vi "3D Experiment Final mouse.vi"() -> ()   [LabVIEW 2011]
uses:
  <vilib>/Utility/miscctls.llb/LV3DPointTypeDef.ctl
  <vilib>/Platform/TimedLoop/XDataNode/timing_clust.ctl
  <vilib>/Platform/TimedLoop/XDataNode/nitl_modes.ctl
  <vilib>/Platform/TimedLoop/XDataNode/wakeup.ctl
  <vilib>/Utility/miscctls.llb/LVRGBAColorTypeDef.ctl
  <vilib>/Utility/inputDevices.llb/closeMouse.vi
  <vilib>/Utility/cursorutil.llb/Set Cursor (Cursor ID).vi
  <vilib>/Utility/inputDevices.llb/mouseAcquire.vi
  <vilib>/Utility/file.llb/Write To Spreadsheet File (DBL).vi
  <vilib>/Utility/file.llb/Write To Spreadsheet File (I64).vi
  <vilib>/Platform/TimedLoop/XDataNode/XDataNode.xnode
  <vilib>/picture/3D Picture Control/NI_3D Picture Control.lvlib
  User32.dll
  <vilib>/Platform/TimedLoop/XDataNode/XDNodeRunTimeDep.lvlib
panel:
  out "initial time 2":u32
  out "initial time":u32
  in  "stop":bool
  out "3D Picture":refnum<vi>(3d-picture)
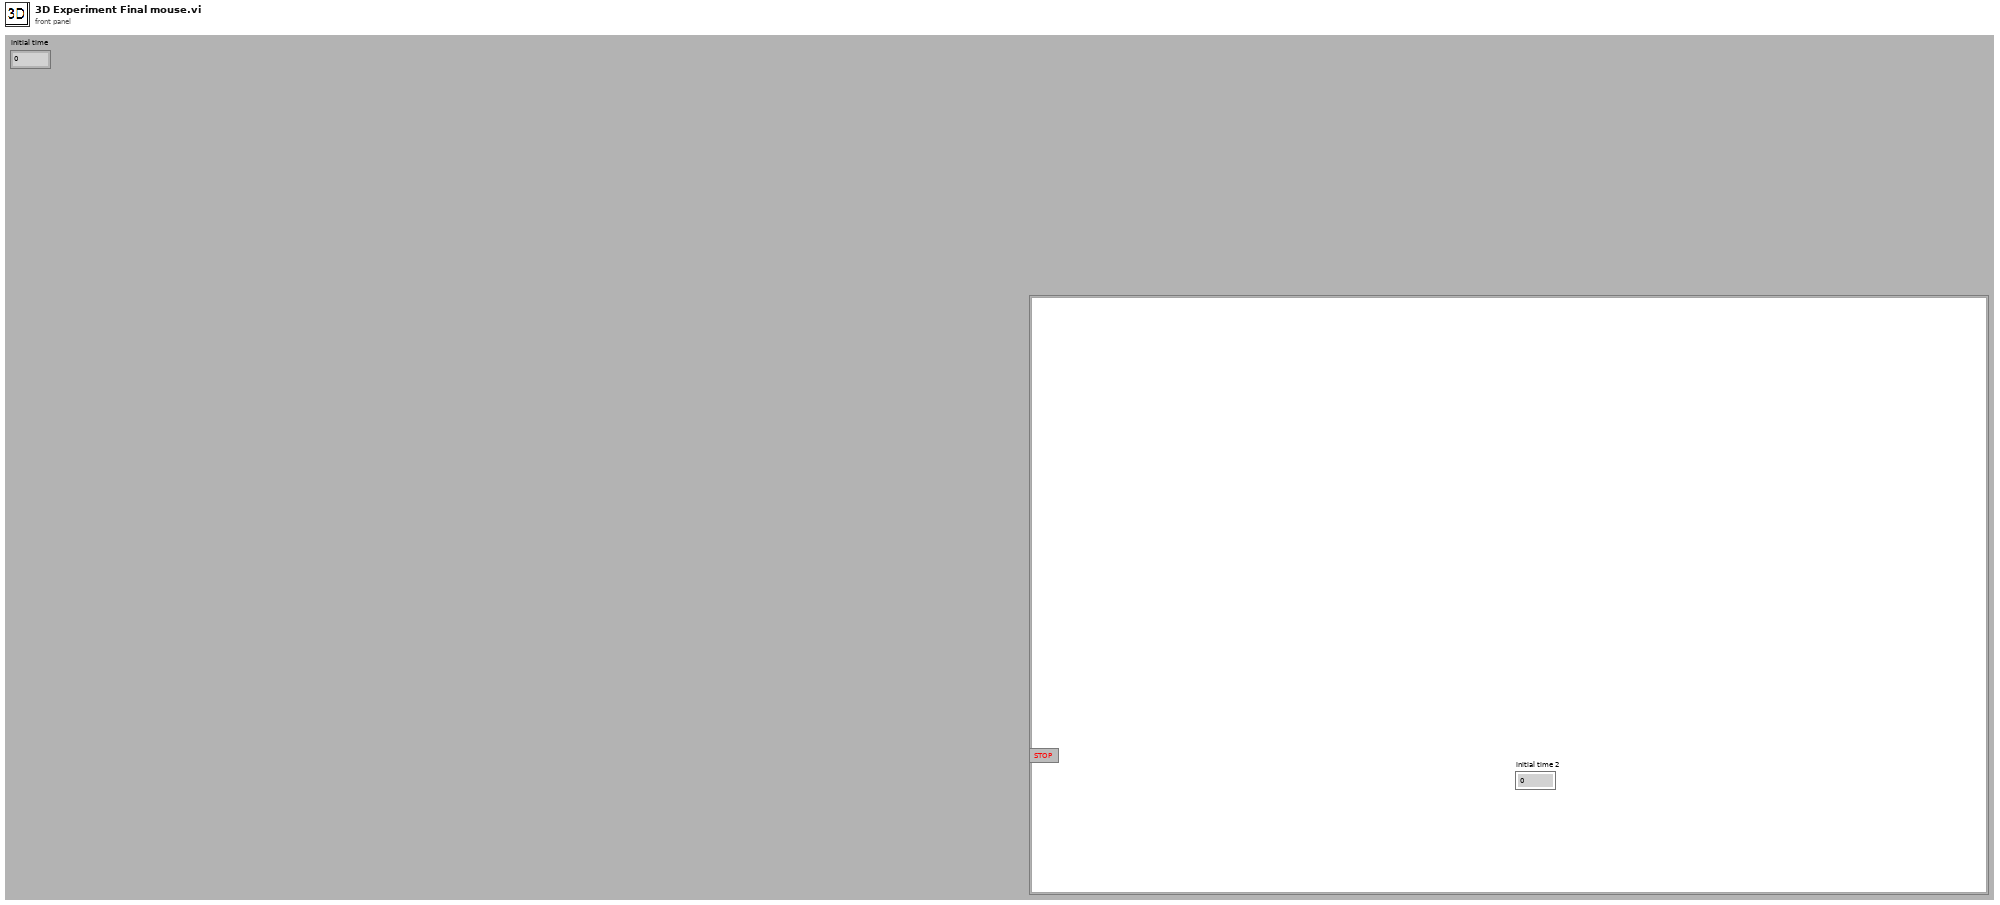
[diagram p1: front panel]
types:
  T1 = enum16{"open", "replace", "create", "open or create", "replace or create", "replace or create with confirmation"}
  T2 = typedef "LV3DPointTypeDef.ctl" = cluster{"X":sgl, "Y":sgl, "Z":sgl}
  T3 = enum16{"Inherit Value", "Points", "Wireframe", "Polygons"}
  T4 = enum16{"Inherit Value", "No Culling", "Cull Back Face", "Cull Front Face", "Cull Both Faces"}
  T5 = enum16{"Zero", "One", "Destination Color", "One Minus Destination Color", "Source Alpha", "One Minus Source Alpha", "Destination Alpha", "One Minus Destination Alpha", "Source Alpha Saturate"}
  T6 = enum16{"Zero", "One", "Source Color", "One Minus Source Color", "Source Alpha", "One Minus Source Alpha", "Destination Alpha", "One Minus Destination Alpha"}
  T7 = enum16{"Normal Bin", "Opaque Bin", "Transparent Bin"}
  T8 = typedef "XDNodeRunTimeDep.lvlib/timing_clust.ctl" = cluster{"Expected End [f-1]":u64, "Actual End [f-1]":u64, "Finished Late? [f-1]":bool, "Expected End [i-1]":u64, "Actual End [i-1]":u64, "Finished Late? [i-1]":bool, "Expected Start [i]":u64, "Actual Start [i]":u64, "Expected Start [f]":u64, "Actual Start [f]":u64, "Source Name":string, "Structure Name":string, "Period":i64, "Deadline":i64, "Offset":i64, "Start":i64, "Priority":i32, "Timeout":i32, "Mode":T9, "Wakeup Reason":T10, "Error":errorcluster, "Source Type":string, "Secondary Source Type":string, "Global End Time":u64, "Global Start Time":u64, "Frame Duration":u64, "Iteration Duration":u64, "Assigned CPU":i32, "I/O Scan Engine Mode":u32}
  T9 = typedef "XDNodeRunTimeDep.lvlib/nitl_modes.ctl" = enum32{"No Change", "Process missed periods, maintain original phase", "Discard missed periods, maintain original phase", "Process missed periods, ignore original phase", "Discard missed periods, ignore original phase"}
  T10 = typedef "XDNodeRunTimeDep.lvlib/wakeup.ctl" = enum32{"Normal", "Aborted", "Asynchronous wakeup", "Timing source error", "Timed loop error", "Timeout"}
  T11 = cluster{"Red":sgl, "Green":sgl, "Blue":sgl, "Alpha":sgl}
  T12 = typedef "LVRGBAColorTypeDef.ctl" = cluster{"Red":sgl, "Green":sgl, "Blue":sgl, "Alpha":sgl}
  T13 = typedef "LVAllMonitorsDisplayTypeDef.ctl" = cluster{"Bounds":cluster{"Left":i16, "Top":i16, "Right":i16, "Bottom":i16}, "Depth":i16}[]
  T14 = cluster{"Bounds":cluster{"Left":i16, "Top":i16, "Right":i16, "Bottom":i16}, "Depth":i16}
  T15 = cluster{"Left":i16, "Top":i16, "Right":i16, "Bottom":i16}
  T16 = cluster{"element":dbl, "Y_scaling":dbl, "element":dbl}
  T17 = cluster{"Horizontal":i32, "Vertical":i32, "Scrolling":i32}
  T18 = cluster{"button 1":bool, "button 2":bool, "button 3":bool, "button 4":bool}
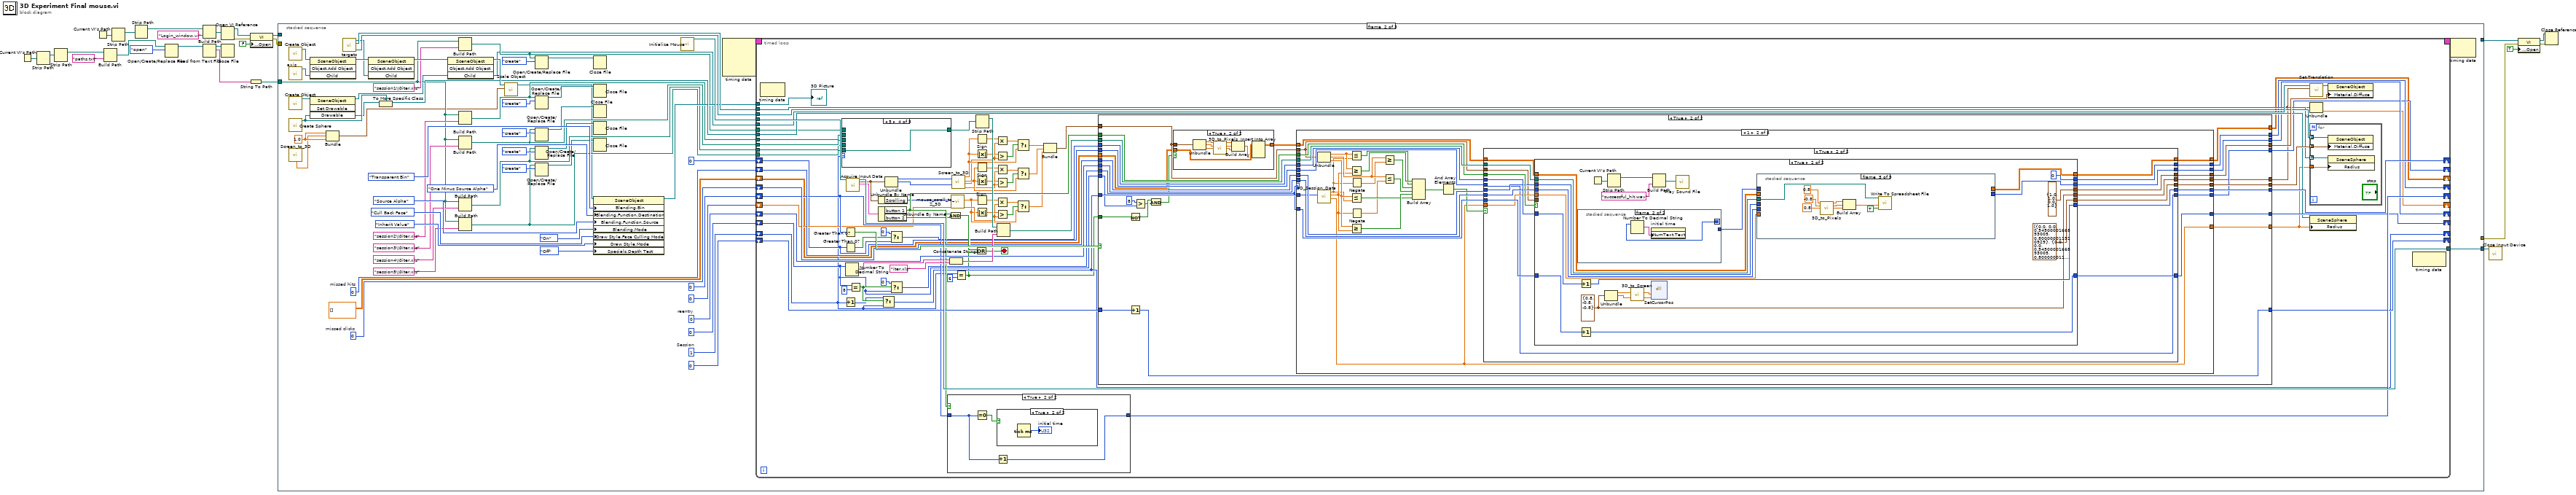
[diagram p0: block diagram]
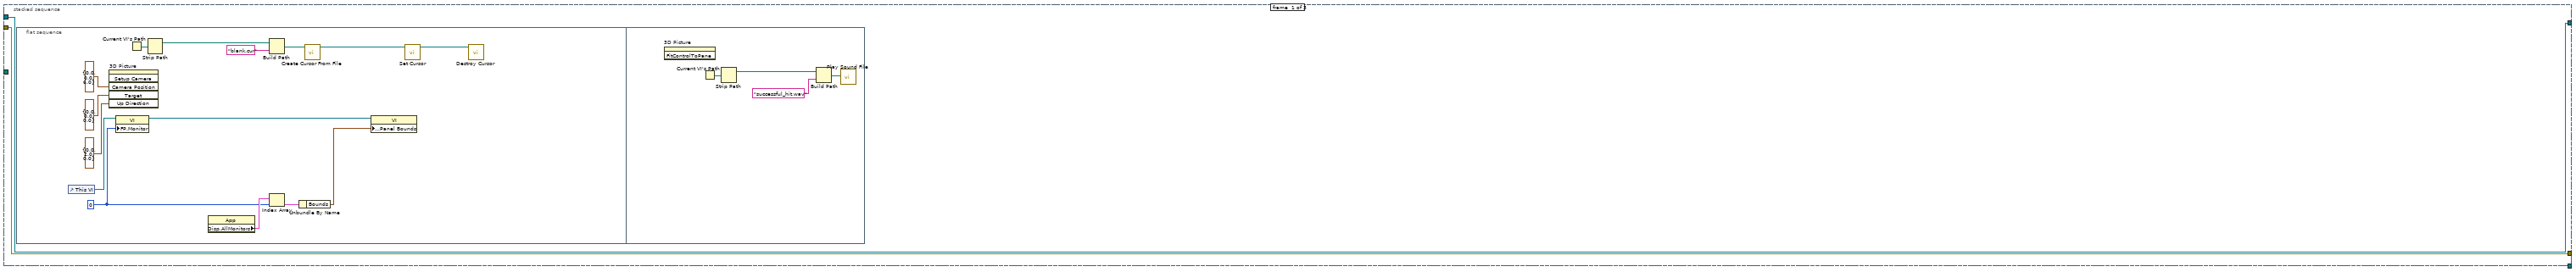
[diagram p2: hidden frame]
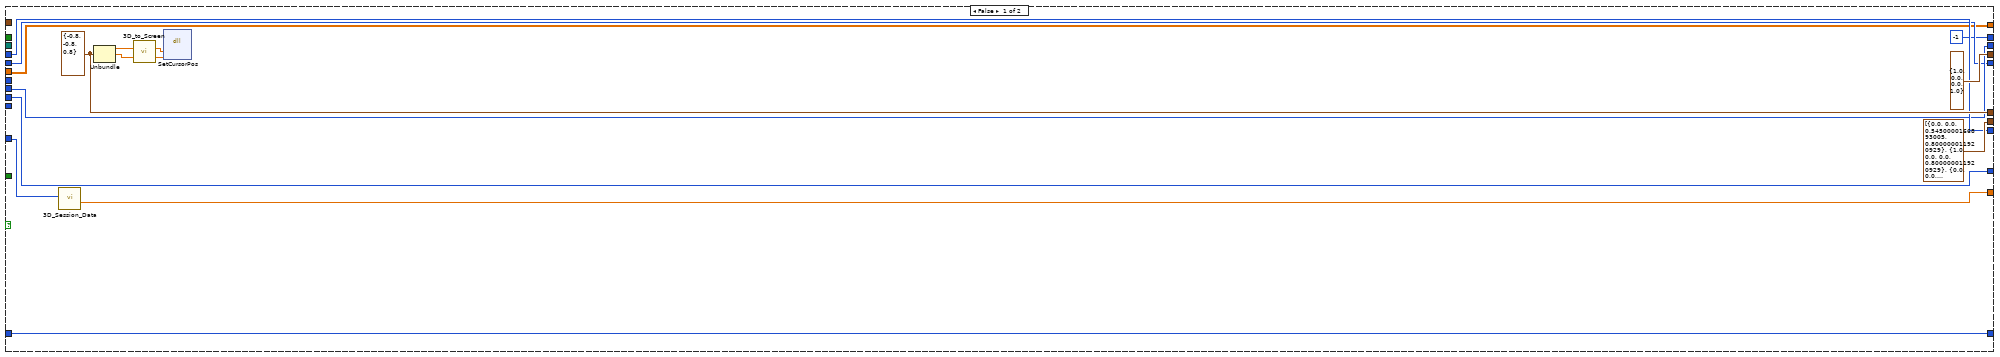
[diagram p7: hidden frame]
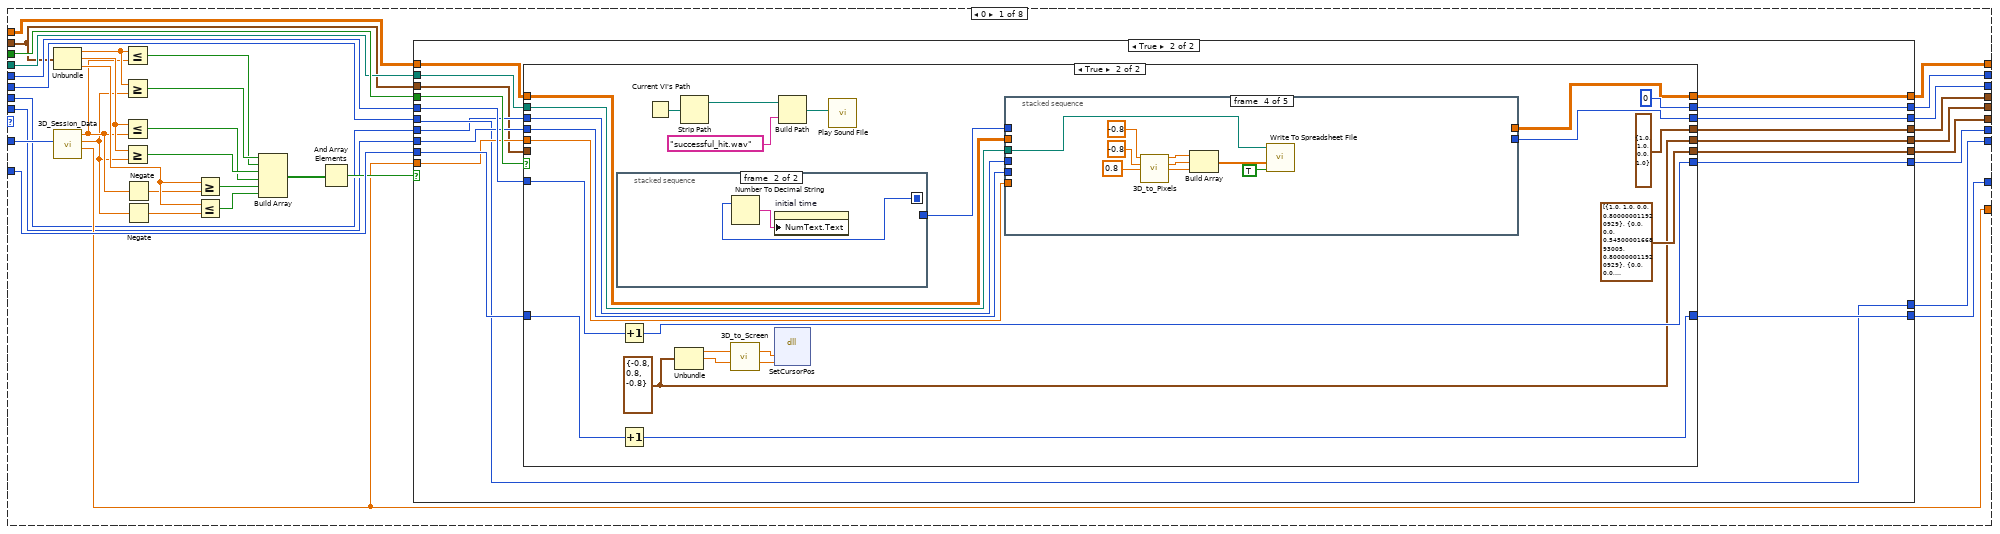
[diagram p9: hidden frame]
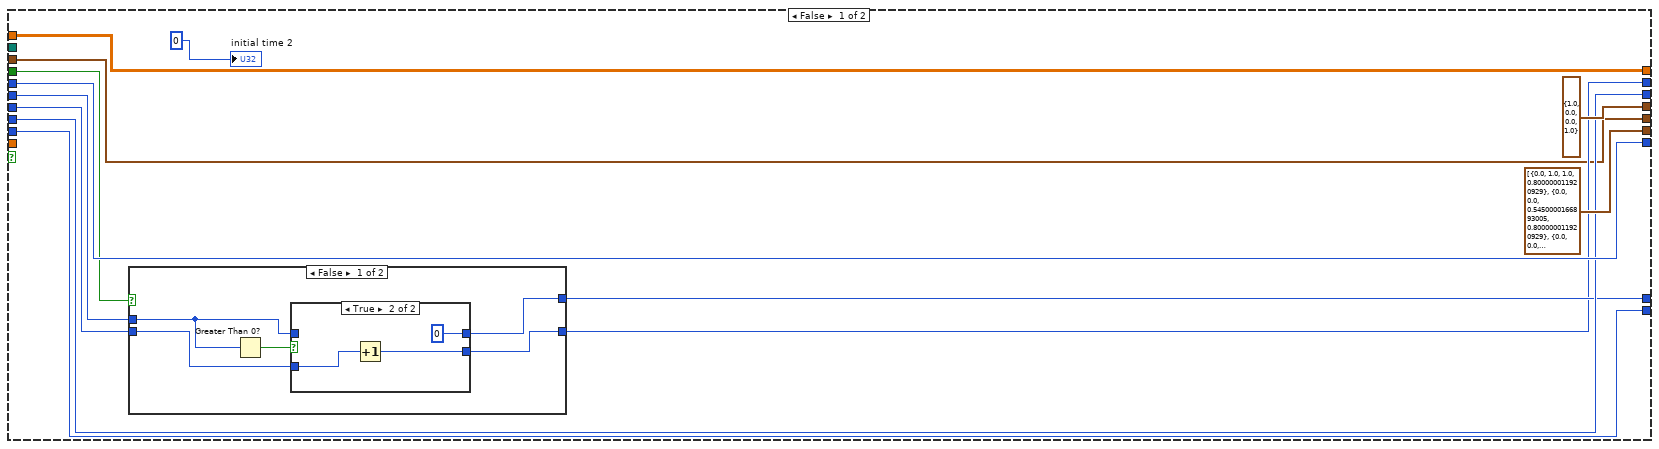
[diagram p10: hidden frame]
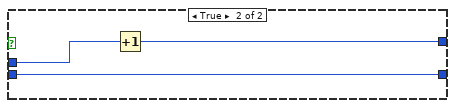
[diagram p12: hidden frame]
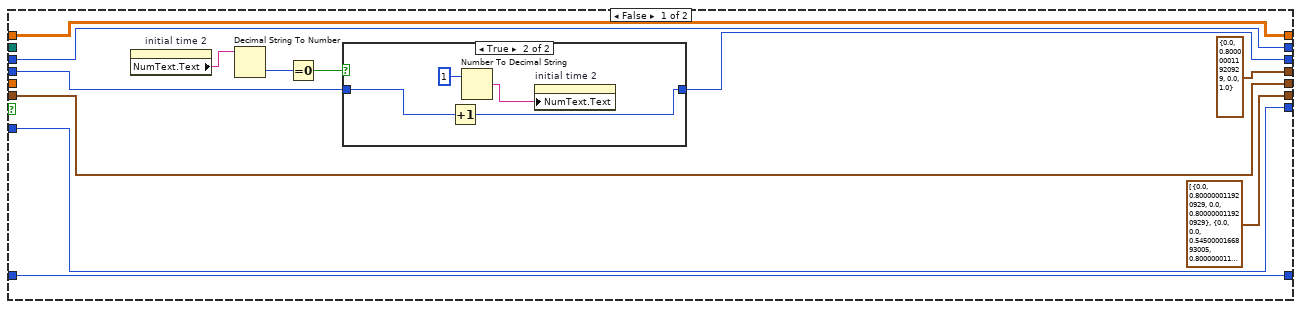
[diagram p13: hidden frame]
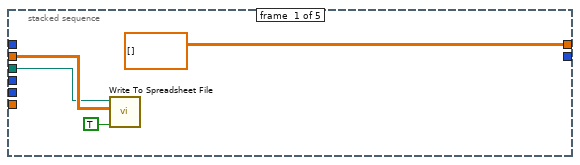
[diagram p15: hidden frame]
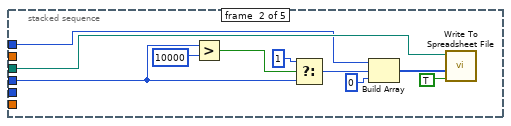
[diagram p16: hidden frame]
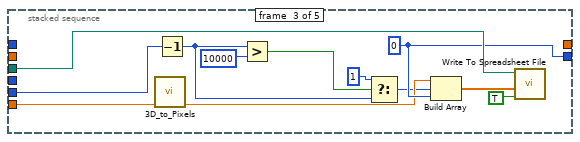
[diagram p17: hidden frame]
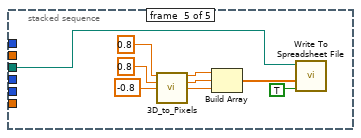
[diagram p18: hidden frame]
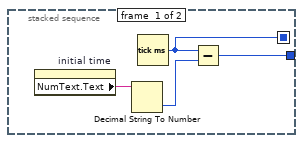
[diagram p19: hidden frame]
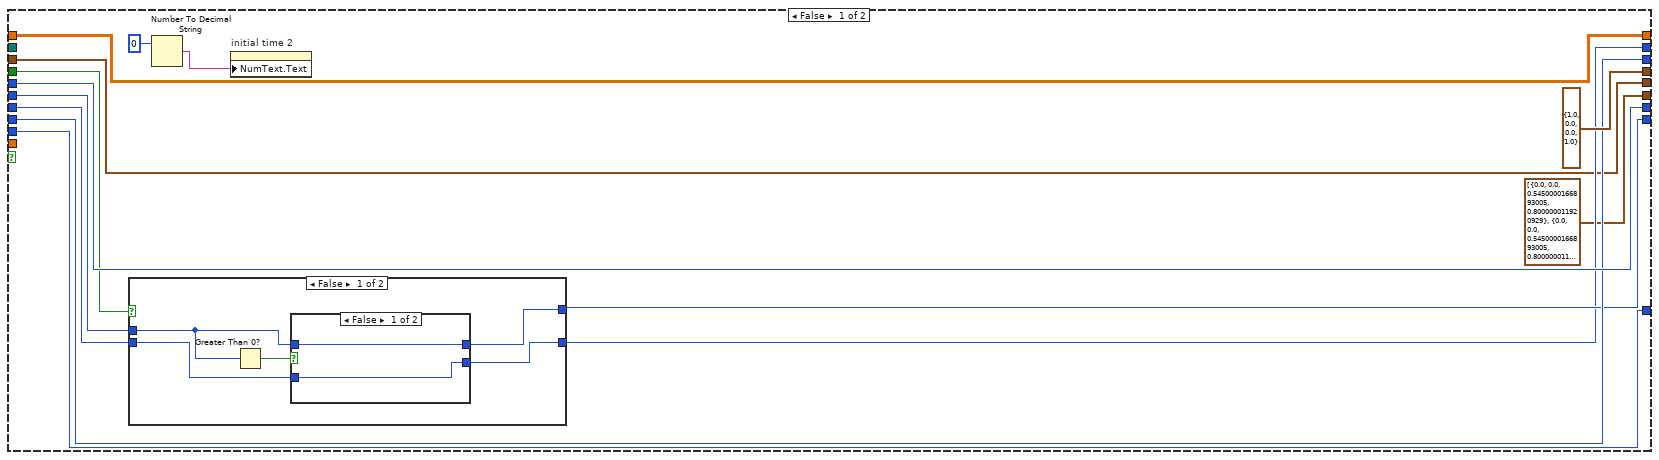
[diagram p20: hidden frame]
diagram:
  n1 = Current VI's Path() -> (path=w1:path)
  n2 = Strip Path(path=w1) -> (stripped path=w2:path)  [unwired: 1 out]
  n3 = Strip Path(path=w2) -> (stripped path=w19:path)  [unwired: 1 out]
  n4 = Current VI's Path() -> (path=w14:path)
  n5 = Build Path(base path=w19, name or relative path="paths.txt") -> (appended path=w22:path)
  n6 = Strip Path(path=w14) -> (stripped path=w11:path)  [unwired: 1 out]
  n7 = Strip Path(path=w11) -> (stripped path=w10:path)  [unwired: 1 out]
  n8 = Open/Create/Replace File(file path (use dialog)=w22, operation (0:open)=T1."open") -> (refnum out=w24:refnum<file>)  [unwired: 4 in, 2 out]
  n9 = Build Path(base path=w10, name or relative path="Login_window.vi") -> (appended path=w12:path)
  n10 = Read from Text File(file (use dialog)=w24) -> (refnum out=w25:refnum<file>, text=w23:string)  [unwired: 3 in, 2 out]
  n11 = Open VI Reference(vi path=w12) -> (vi reference=w17:refnum<vi>, error out=w16:errorcluster)  [unwired: 5 in]
  n12 = Close File(refnum=w25) -> ()  [unwired: 1 in, 2 out]
  n13 = String To Path(string=w23) -> (path=w18:path)
  n14 = property class="VI"(reference=w17, error in=w16, "Front Panel Window:Open"=FALSE) -> (reference out=w9:refnum<vi>, error out=w8:errorcluster)
  n15 = stacked-sequence {
    tunnel: [_ w106 _] -> w26
    tunnel: w18 -> [_ w65 _]
    tunnel: w9 -> [w28 _ _]
    tunnel: w8 -> [w27 _ _]
    tunnel: [w28 _ _] -> w4
    tunnel: [w27 _ _] -> w3
    frame #0 {
      n16 = flat-sequence {
        frame #0 {
          w40 = u16 0 ("Front Panel Window:Monitor")
          n17 = control-ref of="This VI"() -> (w38:refnum<vi>)
          n18 = invoke on="3D Picture" class="SceneGraphDisp (strict)" method="Setup Camera"("Camera Position"=T2 {"X"=0.0, "Y"=0.0, "Z"=6.0}, "Target"=T2 {"X"=0.0, "Y"=0.0, "Z"=0.0}, "Up Direction"=T2 {"X"=0.0, "Y"=2.0, "Z"=0.0}) -> ()  [unwired: 3 in, 6 out]
          n19 = property class="VI"(reference=w38, "FP.Monitor"=w40) -> (reference out=w42:refnum<vi>)  [unwired: 1 in, 1 out]
          n20 = Current VI's Path() -> (path=w37:path)
          n21 = Strip Path(path=w37) -> (stripped path=w36:path)  [unwired: 1 out]
          n22 = property class="App"() -> ("Disp.AllMonitors"=w41:T13)  [unwired: 2 in, 2 out]
          n23 = Build Path(base path=w36, name or relative path="blank.cur") -> (appended path=w34:path)
          n24 = Index Array(array=w41, index=w40) -> (element=w39:T14)
          n25 = Unbundle By Name(w39) -> ("Bounds"=w43:T15)
          n26 = call <vilib>:"Create Cursor From File.vi"("cursor file"=w34) -> ("cursor ID"=w33:refnum<k1>)  [unwired: 9 in, 1 out]
          n27 = property class="VI"(reference=w42, "Front Panel Window:Panel Bounds"=w43) -> ()  [unwired: 1 in, 2 out]
          n28 = call-poly <vilib>:"Set Cursor.vi"("cursor ID"=w33) -> ("previous cursor ID"=w32:refnum<k1>)  [unwired: 9 in, 1 out]
          n29 = call <vilib>:"Destroy Cursor.vi"("cursor ID"=w32) -> ()  [unwired: 9 in, 1 out]
        }
        frame #1 {
          n30 = invoke on="3D Picture" class="SceneGraphDisp (strict)" method="FitControlToPane"() -> ()  [unwired: 3 in, 3 out]
          n31 = Current VI's Path() -> (path=w46:path)
          n32 = Strip Path(path=w46) -> (stripped path=w45:path)  [unwired: 1 out]
          n33 = Build Path(base path=w45, name or relative path="successful_hit.wav") -> (appended path=w47:path)
          n34 = call <vilib>:"Play Sound File.vi"("path"=w47) -> ()  [unwired: 9 in, 2 out]
        }
      }
    }
    frame #1 {
      w52 = 1.0 ("element")
      w53 = 0  # missed clicks
      w54 = 0  # missed hits
      w55 = 0  # reentry
      w94 = 1  # Session
      n35 = call <vilib>:"Create Object.vi"() -> ("Scene:New Object"=w98:refnum<vi>)  [unwired: 10 in, 1 out]
      n36 = call "axis.vi"() -> ("reference out"=w57:refnum<vi>)  [unwired: 11 in]
      n37 = call <vilib>:"Create Object.vi"() -> ("Scene:New Object"=w99:refnum<vi>)  [unwired: 10 in, 1 out]
      n38 = call <vilib>:"Create Sphere.vi"() -> ("New Sphere Refnum"=w92:refnum<vi>)  [unwired: 10 in, 1 out]
      n39 = call "Screen_to_3D.vi"() -> ("Y_scaling"=w49:dbl)  [unwired: 13 in, 6 out]
      n40 = invoke class="SceneObject" method="Object.Add Object"(reference=w98, "Child"=w57) -> (reference out=w97:refnum<vi>)  [unwired: 2 in, 3 out]
      n41 = invoke class="SceneObject" method="Set Drawable"(reference=w99, "Drawable"=w92) -> (reference out=w58:refnum<vi>, "Drawable"=w91:refnum<vi>)  [unwired: 2 in, 2 out]
      n42 = Bundle("element"=w52, "Y_scaling"=w49, "element"=w52) -> (w51:T16)  [unwired: 1 in]
      n43 = call "targets.vi"() -> ("objects"=w93:refnum<vi>[], "shperes"=w89:refnum<vi>[], "Scene:New Object"=w56:refnum<vi>)  [unwired: 8 in]
      n44 = invoke class="SceneObject" method="Object.Add Object"(reference=w97, "Child"=w56) -> (reference out=w96:refnum<vi>)  [unwired: 2 in, 3 out]
      n45 = To More Specific Class(target class=w92, reference=w91) -> (specific class reference=w90:refnum<vi>)  [unwired: 1 in, 1 out]
      n46 = invoke class="SceneObject" method="Object.Add Object"(reference=w96, "Child"=w58) -> (reference out=w95:refnum<vi>, "Child"=w59:refnum<vi>)  [unwired: 2 in, 2 out]
      n47 = Build Path(base path=w65, name or relative path="session1\\0iter.xls") -> (appended path=w60:path)
      n48 = Build Path(base path=w65, name or relative path="session2\\0iter.xls") -> (appended path=w61:path)
      n49 = Build Path(base path=w65, name or relative path="session3\\0iter.xls") -> (appended path=w63:path)
      n50 = Build Path(base path=w65, name or relative path="session4\\0iter.xls") -> (appended path=w62:path)
      n51 = Build Path(base path=w65, name or relative path="session5\\0iter.xls") -> (appended path=w64:path)
      n52 = call <vilib>:"Scale Object.vi"("Scale"=w51, "Scene.Object In"=w95) -> ("Scene.Object Out"=w50:refnum<vi>)  [unwired: 8 in, 1 out]
      n53 = Open/Create/Replace File(file path (use dialog)=w60, operation (0:open)=T1."create") -> (refnum out=w73:refnum<file>)  [unwired: 4 in, 2 out]
      n54 = Open/Create/Replace File(file path (use dialog)=w61, operation (0:open)=T1."create") -> (refnum out=w75:refnum<file>)  [unwired: 4 in, 2 out]
      n55 = Open/Create/Replace File(file path (use dialog)=w63, operation (0:open)=T1."create") -> (refnum out=w70:refnum<file>)  [unwired: 4 in, 2 out]
      n56 = Open/Create/Replace File(file path (use dialog)=w62, operation (0:open)=T1."create") -> (refnum out=w67:refnum<file>)  [unwired: 4 in, 2 out]
      n57 = Open/Create/Replace File(file path (use dialog)=w64, operation (0:open)=T1."create") -> (refnum out=w68:refnum<file>)  [unwired: 4 in, 2 out]
      n58 = Close File(refnum=w73) -> ()  [unwired: 1 in, 2 out]
      n59 = Close File(refnum=w75) -> ()  [unwired: 1 in, 2 out]
      n60 = Close File(refnum=w70) -> ()  [unwired: 1 in, 2 out]
      n61 = Close File(refnum=w67) -> ()  [unwired: 1 in, 2 out]
      n62 = Close File(refnum=w68) -> ()  [unwired: 1 in, 2 out]
      n63 = property class="SceneObject"(reference=w50, "Blending.Bin"=T7."Transparent Bin" ("Blending:Bin"), "Blending.Function.Destination"=T6."One Minus Source Alpha" ("Blending:Function:Destination"), "Blending.Function.Source"=T5."Source Alpha" ("Blending:Function:Source"), "Blending.Mode"=enum16{"Inherit Value", "Off", "On"}."On" ("Blending:Mode"), "Draw Style.Face Culling Mode"=T4."Cull Back Face" ("Draw Style:Face Culling Mode"), "Draw Style.Mode"=T3."Inherit Value" ("Draw Style:Mode"), "Specials.Depth Test"=enum16{"Inherit Value", "Off", "On"}."Off" ("Specials:Depth Test")) -> (reference out=w81:refnum<vi>)  [unwired: 1 in, 1 out]
      n64 = call <vilib>:"Initialize Mouse.vi"() -> ("device ID"=w105:refnum<k1>)  [unwired: 1 in, 10 out]
      n65 = node-c288() -> (w108:T8)  [unwired: 4 in]
      n66 = timed-loop {
        tunnel: [w193] -> w106
        tunnel: w105 -> [w192]
        shift-right: [w191] -> _
        shift-left: 0 ("y") -> [w153]
        shift-right: [w188] -> _
        shift-left: 0 ("y") -> [w137]
        shift-right: [w118] -> _
        shift-left: 0 ("x") -> [w146]
        shift-right: [w186] -> _
        shift-left: 0 ("y") -> [w142]
        timing: w108 -> [_]
        timing-out: [_] -> w107
        shift-right: [w117] -> _
        shift-left: w94 -> [w116]
        shift-right: [w182] -> _
        shift-left: 0 ("y") -> [w183]
        tunnel: w81 -> [w181]
        tunnel: w59 -> [w180]
        tunnel: w93 -> [w177]
        tunnel: w90 -> [w175]
        tunnel: w89 -> [w173]
        tunnel: w64 -> [w169]
        tunnel: w63 -> [w168]
        tunnel: w62 -> [w167]
        tunnel: w61 -> [w166]
        tunnel: w60 -> [w165]
        shift-right: [w160] -> _
        shift-left: w55 -> [w161]
        shift-right: [w154] -> _
        shift-left: w54 -> [w157]
        shift-right: [w155] -> _
        shift-left: w53 -> [w156]
        shift-right: [w113] -> _
        shift-left: dbl[][] [] -> [w114]
        stop <- w158 stop-if-true
        n67 = node-c288() -> ()  [unwired: 1 in, 1 out]
        n68 = case shown="5" w116 {
          tunnel: w169 -> [_ _ _ w197 _]
          tunnel: w167 -> [_ _ w196 _ _]
          tunnel: w168 -> [_ w195 _ _ _]
          tunnel: w166 -> [w194 _ _ _ _]
          tunnel: w165 -> [_ _ _ _ w198]
          tunnel: [w194 w195 w196 w197 w198] -> w162
          frame 2 {
          }
          frame 3 {
          }
          frame 4 {
          }
          frame 5 {
          }
          frame 1, Default {
          }
        }
        n69 = Greater Than 0?(x=w153) -> (x > 0?=w190:bool)
        n70 = Greater Than 0?(x=w142) -> (x > 0?=w145:bool)
        n71 = Increment(x=w116) -> (x+1=w138:i32)
        n72 = Number To Decimal String(number=w137) -> (decimal integer string=w170:string)  [unwired: 1 in]
        n73 = call-poly <vilib>:"Acquire Input Data.vi"("device ID"=w192) -> ("device ID"=w193:refnum<k1>, "axis info"=w187:T17, "button info"=w189:T18)  [unwired: 2 in, 14 out]
        n74 = Equal?(x=w137, y=8) -> (x = y?=w141:bool)
        n75 = Unbundle By Name(w187) -> ("Scrolling"=w147:i32)
        n76 = Unbundle By Name(w189) -> ("button 1"=w152:bool, "button 2"=w151:bool)
        n77 = Select(t=w138, s=w141, f=w116) -> (s? t:f=w117:i32)
        n78 = Unbundle(w187) -> ("Horizontal"=w149:i32, "Vertical"=w148:i32)  [unwired: 1 out]
        n79 = Select(t=0 ("y"), s=w145, f=w142) -> (s? t:f=w143:i32)
        n80 = Select(t=0 ("y"), s=w141, f=w137) -> (s? t:f=w139:i32)
        n81 = case shown="True" w152 {
          tunnel: w153 -> [w1626 w1627]
          tunnel: [w1626 w1629] -> w191
          frame False {
          }
          frame True {
            n82 = Equal To 0?(x=w1627) -> (x = 0?=w1628:bool)
            n83 = Increment(x=w1627) -> (x+1=w1629:i32)
            n84 = case shown="True" w1628 {
              frame False {
              }
              frame True {
                n85 = Tick Count (ms)() -> (millisecond timer value=→"initial time":u32)
              }
            }
          }
        }
        n86 = And(x=w152, y=w151) -> (x .and. y?=w159:bool)
        n87 = Concatenate Strings(w170, "iter.xls" ("name or relative path")) -> (w171:string)
        n88 = call "mouse_scroll_to_Z_3D.vi"("Previous_Z"=w146, "Scrolling"=w147) -> ("Zmax"=w132:dbl, "Z"=w112:dbl)  [unwired: 8 in]
        n89 = call "Screen_to_3D.vi"("X"=w149, "Y"=w148) -> ("X_3D"=w127:dbl, "Y_3D"=w122:dbl, "Xmax"=w120:dbl, "Ymax"=w121:dbl)  [unwired: 11 in, 3 out]
        n90 = Equal?(x=w116, y=6) -> (x = y?=w115:bool)
        n91 = Or(x=w159, y=w115) -> (x .or. y?=w158:bool)
        n92 = Sign(1:w127) -> (0:w129:dbl)
        n93 = Absolute Value(x=w127) -> (abs(x)=w130:dbl)
        n94 = Sign(1:w122) -> (0:w124:dbl)
        n95 = Absolute Value(x=w122) -> (abs(x)=w125:dbl)
        n96 = Sign(1:w112) -> (0:w134:dbl)
        n97 = Absolute Value(x=w112) -> (abs(x)=w135:dbl)
        n98 = Strip Path(path=w162) -> (stripped path=w163:path)  [unwired: 1 out]
        n99 = Multiply(x=w129, y=w120) -> (x*y=w128:dbl)
        n100 = Greater?(x=w130, y=w120) -> (0:w131:bool)
        n101 = Multiply(x=w124, y=w121) -> (x*y=w123:dbl)
        n102 = Greater?(x=w125, y=w121) -> (0:w126:bool)
        n103 = Multiply(x=w134, y=w132) -> (x*y=w133:dbl)
        n104 = Greater?(x=w135, y=w132) -> (0:w136:bool)
        n105 = Build Path(base path=w163, name or relative path=w171) -> (appended path=w164:path)
        n106 = Select(t=w128, s=w131, f=w127) -> (s? t:f=w110:dbl)
        n107 = Select(t=w123, s=w126, f=w122) -> (s? t:f=w109:dbl)
        n108 = Select(t=w133, s=w136, f=w112) -> (s? t:f=w111:dbl)
        n109 = Bundle("X_3D"=w110, "Y_3D"=w109, "Z"=w111) -> (w150:cluster{"X_3D":dbl, "Y_3D":dbl, "Z":dbl})  [unwired: 1 in]
        n110 = case shown="True" w190 {
          tunnel: w150 -> [_ w230]
          tunnel: [w217 w231] -> w119
          tunnel: [T12[] [{"Red"=0.0, "Green"=0.0, "Blue"=0.545, "Alpha"=0.8}, {"Red"=1.0, "Green"=0.0, "Blue"=0.0, "Alpha"=0.8}, {"Red"=0.0, "Green"=0.0, "Blue"=0.545, "Alpha"=0.8}, {"Red"=0.0, "Green"=0.0, "Blue"=0.545, "Alpha"=0.8}, {"Red"=0.0, "Green"=0.0, "Blue"=0.545, "Alpha"=0.8}, {"Red"=0.0, "Green"=0.0, "Blue"=0.545, "Alpha"=0.8}, {"Red"=0.0, "Green"=0.0, "Blue"=0.545, "Alpha"=0.8}, {"Red"=0.0, "Green"=0.0, "Blue"=0.545, "Alpha"=0.8}] ("Array") w249] -> w176
          tunnel: w139 -> [w218 w228]
          tunnel: w152 -> [_ w247]
          tunnel: [T11 {"Red"=1.0, "Green"=0.0, "Blue"=0.0, "Alpha"=1.0} ("Color") w248] -> w179
          tunnel: [w218 w246] -> w188
          tunnel: w143 -> [w216 w245]
          tunnel: [w216 w244] -> w186
          tunnel: w117 -> [w214 w243]
          tunnel: w183 -> [w215 w242]
          tunnel: [w215 w241] -> w182
          tunnel: [w213 w240] -> w174
          tunnel: w164 -> [_ w236]
          tunnel: w161 -> [w212 w239]
          tunnel: [w212 w238] -> w160
          tunnel: w137 -> [_ w237]
          tunnel: w157 -> [w211 w235]
          tunnel: w156 -> [_ w234]
          tunnel: [-1 ("y") w233] -> w155
          tunnel: [w211 w232] -> w154
          tunnel: w115 -> [_ w227]
          tunnel: w114 -> [w205 w223]
          tunnel: [w205 w221] -> w113
          frame False {
            w217 = cluster{dbl, dbl, "y":dbl} {-0.8, -0.8, "y"=0.8}
            n111 = call "3D_Session_Data.vi"("Session"=w214) -> ("Radius"=w213:sgl)  [unwired: 8 in, 2 out]
            n112 = Unbundle(w217) -> (w210:dbl, w209:dbl)  [unwired: 1 out]
            n113 = call "3D_to_Screen.vi"("X_3D"=w210, "Y_3D"=w209) -> ("X"=w208:dbl, "Y"=w207:dbl)  [unwired: 11 in, 1 out]
            n114 = dll-call lib="User32.dll" fn="SetCursorPos"(w208, w207) -> ()  [unwired: 6 in, 2 out]
          }
          frame True {
            n115 = Not(x=w227) -> (.not. x?=w226:bool)
            n116 = Increment(x=w242) -> (x+1=w241:i32)
            n117 = Greater?(x=8 ("y"), y=w237) -> (0:w225:bool)
            n118 = And(x=w226, y=w225) -> (x .and. y?=w224:bool)
            n119 = case shown="True" w224 {
              tunnel: w230 -> [_ w260]
              tunnel: w223 -> [w250 w253]
              tunnel: [w250 w251] -> w222
              frame False {
              }
              frame True {
                n120 = Unbundle(w260) -> ("X_3D"=w259:dbl, "Y_3D"=w258:dbl, "Z"=w257:dbl)
                n121 = call "3D_to_Pixels.vi"("X_3D"=w259, "Y_3D"=w258, "Z_3D"=w257) -> ("X_pixels"=w256:dbl, "Y_pixels"=w255:dbl, "Z_pixels"=w254:dbl)  [unwired: 9 in, 1 out]
                n122 = Build Array(w256, w255, w254) -> (w252:dbl[])
                n123 = Insert Into Array(array=w253, new element=w252) -> (w251:dbl[][])  [unwired: 2 in]
              }
            }
            n124 = case shown="1" w228 {
              tunnel: [w295 w465 w636 w807 w976 w1147 w1318 w1489] -> w249
              tunnel: w230 -> [w264 w433 w604 w775 w945 w1115 w1285 w1457]
              tunnel: [w294 w464 w635 w806 w975 w1146 w1317 w1488] -> w248
              tunnel: w247 -> [w293 w452 w634 w805 w974 w1145 w1316 w1487]
              tunnel: w228 -> [w292 w463 w633 w804 w973 w1144 w1315 w1486]
              tunnel: [w291 w462 w632 w803 w972 w1143 w1314 w1485] -> w246
              tunnel: w245 -> [w279 w461 w631 w802 w971 w1142 w1313 w1484]
              tunnel: [w278 w460 w630 w801 w970 w1141 w1312 w1483] -> w244
              tunnel: w243 -> [w277 w432 w603 w773 w946 w1114 w1286 w1456]
              tunnel: [w271 w431 w602 w776 w944 w1113 w1284 w1455] -> w240
              tunnel: w236 -> [w272 w459 w629 w800 w969 w1140 w1311 w1482]
              tunnel: w239 -> [w269 w457 w627 w798 w967 w1138 w1309 w1481]
              tunnel: [w270 w458 w628 w799 w968 w1139 w1310 w1480] -> w238
              tunnel: w235 -> [w268 w456 w626 w797 w966 w1137 w1308 w1479]
              tunnel: w234 -> [w267 w455 w625 w796 w965 w1136 w1307 w1478]
              tunnel: [w265 w453 w623 w794 w963 w1134 w1305 w1477] -> w233
              tunnel: [w266 w454 w624 w795 w964 w1135 w1306 w1476] -> w232
              tunnel: [w263 w451 w622 w793 w962 w1133 w1304 w1475] -> w231
              tunnel: w222 -> [w262 w449 w621 w792 w961 w1132 w1303 w1474]
              tunnel: [w261 w450 w620 w791 w960 w1131 w1302 w1473] -> w221
              frame 0 {
                n125 = Unbundle(w264) -> ("X_3D"=w290:dbl, "Y_3D"=w289:dbl, "Z"=w288:dbl)
                n126 = call "3D_Session_Data.vi"("Session"=w277) -> ("Radius"=w271:sgl, "min"=w275:dbl, "max"=w276:dbl)  [unwired: 8 in]
                n127 = Less Or Equal?(x=w290, y=w276) -> (x <= y?=w286:bool)
                n128 = Greater Or Equal?(x=w290, y=w275) -> (x >= y?=w287:bool)
                n129 = Less Or Equal?(x=w289, y=w276) -> (x <= y?=w284:bool)
                n130 = Greater Or Equal?(x=w289, y=w275) -> (x >= y?=w285:bool)
                n131 = Negate(x=w276) -> (-x=w274:dbl)
                n132 = Negate(x=w275) -> (-x=w273:dbl)
                n133 = Greater Or Equal?(x=w288, y=w274) -> (x >= y?=w283:bool)
                n134 = Less Or Equal?(x=w288, y=w273) -> (x <= y?=w282:bool)
                n135 = Build Array(w287, w286, w285, w284, w283, w282) -> (w281:bool[])
                n136 = And Array Elements(Boolean array=w281) -> (logical AND=w280:bool)
                n137 = case shown="True" w280 {
                  tunnel: [T12[] [{"Red"=0.0, "Green"=1.0, "Blue"=1.0, "Alpha"=0.8}, {"Red"=0.0, "Green"=0.0, "Blue"=0.545, "Alpha"=0.8}, {"Red"=0.0, "Green"=0.0, "Blue"=0.545, "Alpha"=0.8}, {"Red"=0.0, "Green"=0.0, "Blue"=0.545, "Alpha"=0.8}, {"Red"=0.0, "Green"=0.0, "Blue"=0.545, "Alpha"=0.8}, {"Red"=0.0, "Green"=0.0, "Blue"=0.545, "Alpha"=0.8}, {"Red"=0.0, "Green"=0.0, "Blue"=0.545, "Alpha"=0.8}, {"Red"=0.0, "Green"=0.0, "Blue"=0.545, "Alpha"=0.8}] ("Array") w339] -> w295
                  tunnel: [T11 {"Red"=1.0, "Green"=0.0, "Blue"=0.0, "Alpha"=1.0} ("Color") w338] -> w294
                  tunnel: w293 -> [w298 w337]
                  tunnel: w292 -> [w306 w336]
                  tunnel: [w306 w335] -> w291
                  tunnel: w279 -> [w305 w334]
                  tunnel: [w305 w333] -> w278
                  tunnel: w272 -> [_ w332]
                  tunnel: w271 -> [_ w331]
                  tunnel: [w304 w330] -> w270
                  tunnel: w269 -> [w304 w329]
                  tunnel: w268 -> [w302 w328]
                  tunnel: w267 -> [w301 w327]
                  tunnel: [w300 w328] -> w266
                  tunnel: [w299 w326] -> w265
                  tunnel: w264 -> [w297 w325]
                  tunnel: [w297 w324] -> w263
                  tunnel: w262 -> [w296 w323]
                  tunnel: [w296 w322] -> w261
                  frame False {
                    n138 = case shown="False" w298 {
                      tunnel: w302 -> [w309 w321]
                      tunnel: [w310 w320] -> w300
                      tunnel: w301 -> [w312 w319]
                      tunnel: [w311 w319] -> w299
                      frame False {
                        n139 = Greater Than 0?(x=w309) -> (x > 0?=w313:bool)
                        n140 = case shown="True" w313 {
                          tunnel: w312 -> [w315 w318]
                          tunnel: [w315 w317] -> w311
                          tunnel: w309 -> [w314 _]
                          tunnel: [w314 0 ("y")] -> w310
                          frame False {
                          }
                          frame True {
                            n141 = Increment(x=w318) -> (x+1=w317:i32)
                          }
                        }
                      }
                      frame True {
                        n142 = Increment(x=w321) -> (x+1=w320:i32)
                      }
                    }
                    "initial time 2" <- u32 0 ("initial time 2")
                  }
                  frame True {
                    n143 = case shown="True" w337 {
                      tunnel: [T12[] [{"Red"=0.0, "Green"=0.8, "Blue"=0.0, "Alpha"=0.8}, {"Red"=0.0, "Green"=0.0, "Blue"=0.545, "Alpha"=0.8}, {"Red"=0.0, "Green"=0.0, "Blue"=0.545, "Alpha"=0.8}, {"Red"=0.0, "Green"=0.0, "Blue"=0.545, "Alpha"=0.8}, {"Red"=0.0, "Green"=0.0, "Blue"=0.545, "Alpha"=0.8}, {"Red"=0.0, "Green"=0.0, "Blue"=0.545, "Alpha"=0.8}, {"Red"=0.0, "Green"=0.0, "Blue"=0.545, "Alpha"=0.8}, {"Red"=0.0, "Green"=0.0, "Blue"=0.545, "Alpha"=0.8}] ("Array") T12[] [{"Red"=1.0, "Green"=1.0, "Blue"=0.0, "Alpha"=0.8}, {"Red"=0.0, "Green"=0.0, "Blue"=0.545, "Alpha"=0.8}, {"Red"=0.0, "Green"=0.0, "Blue"=0.545, "Alpha"=0.8}, {"Red"=0.0, "Green"=0.0, "Blue"=0.545, "Alpha"=0.8}, {"Red"=0.0, "Green"=0.0, "Blue"=0.545, "Alpha"=0.8}, {"Red"=0.0, "Green"=0.0, "Blue"=0.545, "Alpha"=0.8}, {"Red"=0.0, "Green"=0.0, "Blue"=0.545, "Alpha"=0.8}, {"Red"=0.0, "Green"=0.0, "Blue"=0.545, "Alpha"=0.8}] ("Array")] -> w339
                      tunnel: [T11 {"Red"=0.0, "Green"=0.8, "Blue"=0.0, "Alpha"=1.0} ("Color") T11 {"Red"=1.0, "Green"=1.0, "Blue"=0.0, "Alpha"=1.0} ("Color")] -> w338
                      tunnel: w336 -> [w349 w378]
                      tunnel: [w349 w377] -> w335
                      tunnel: w334 -> [w348 w360]
                      tunnel: [w348 w376] -> w333
                      tunnel: w332 -> [_ w370]
                      tunnel: w331 -> [_ w369]
                      tunnel: [w343 w368] -> w330
                      tunnel: w329 -> [w344 w367]
                      tunnel: w327 -> [w342 w366]
                      tunnel: [w342 0 ("x")] -> w326
                      tunnel: w325 -> [w341 _]
                      tunnel: [w341 w359] -> w324
                      tunnel: w323 -> [w340 w358]
                      tunnel: [w340 w357] -> w322
                      frame False {
                        n144 = property on="initial time 2" class="DigNum (strict)"() -> ("NumText.Text"=w346:string)  [unwired: 2 in, 2 out]
                        n145 = Decimal String To Number(string=w346) -> (number=w345:i32)  [unwired: 2 in, 1 out]
                        n146 = Equal To 0?(x=w345) -> (x = 0?=w347:bool)
                        n147 = case shown="True" w347 {
                          tunnel: w344 -> [w352 w356]
                          tunnel: [w352 w355] -> w343
                          frame False {
                          }
                          frame True {
                            n148 = Increment(x=w356) -> (x+1=w355:u32)
                            n149 = Number To Decimal String(number=1) -> (decimal integer string=w354:string)  [unwired: 1 in]
                            n150 = property on="initial time 2" class="DigNum (strict)"("NumText.Text"=w354) -> ()  [unwired: 2 in, 2 out]
                          }
                        }
                      }
                      frame True {
                        w359 = cluster{dbl, dbl, "y":dbl} {-0.8, 0.8, "y"=-0.8}
                        n151 = stacked-sequence {
                          seq-local: [w426 _] -> [_ w429]
                          tunnel: [w425 _] -> w371
                          frame #0 {
                            n152 = property on="initial time" class="DigNum (strict)"() -> ("NumText.Text"=w428:string)  [unwired: 2 in, 2 out]
                            n153 = Decimal String To Number(string=w428) -> (number=w427:i32)  [unwired: 2 in, 1 out]
                            n154 = Tick Count (ms)() -> (millisecond timer value=w426:u32)
                            n155 = Subtract(x=w426, y=w427) -> (x-y=w425:u32)
                          }
                          frame #1 {
                            n156 = Number To Decimal String(number=w429) -> (decimal integer string=w430:string)  [unwired: 1 in]
                            n157 = property on="initial time" class="DigNum (strict)"("NumText.Text"=w430) -> ()  [unwired: 2 in, 2 out]
                          }
                        }
                        n158 = Increment(x=w360) -> (x+1=w376:i32)
                        n159 = Increment(x=w378) -> (x+1=w377:i32)
                        n160 = Current VI's Path() -> (path=w374:path)
                        n161 = Unbundle(w359) -> (w364:dbl, w365:dbl)  [unwired: 1 out]
                        n162 = Strip Path(path=w374) -> (stripped path=w373:path)  [unwired: 1 out]
                        n163 = call "3D_to_Screen.vi"("X_3D"=w364, "Y_3D"=w365) -> ("X"=w363:dbl, "Y"=w362:dbl)  [unwired: 11 in, 1 out]
                        n164 = dll-call lib="User32.dll" fn="SetCursorPos"(w363, w362) -> ()  [unwired: 6 in, 2 out]
                        n165 = Build Path(base path=w373, name or relative path="successful_hit.wav") -> (appended path=w375:path)
                        n166 = call <vilib>:"Play Sound File.vi"("path"=w375) -> ()  [unwired: 9 in, 2 out]
                        n167 = stacked-sequence {
                          tunnel: w370 -> [w381 w393 w404 w414 w423]
                          tunnel: w371 -> [_ w391 _ _ _]
                          tunnel: w369 -> [_ _ w401 _ _]
                          tunnel: [_ _ w402 _ _] -> w368
                          tunnel: w367 -> [_ _ w403 _ _]
                          tunnel: w366 -> [_ w387 _ _ _]
                          tunnel: w358 -> [w383 _ _ _ _]
                          tunnel: [dbl[][] [] _ _ _ _] -> w357
                          frame #0 {
                            n168 = call-poly <vilib>:"Write To Spreadsheet File.vi"("append to file? (new file:F)"=TRUE, "2D data"=w383, "file path (dialog if empty)"=w381) -> ()  [unwired: 5 in, 1 out]
                          }
                          frame #1 {
                            n169 = Greater?(x=w387, y=u32 10000 ("element")) -> (0:w389:bool)
                            n170 = Select(t=1, s=w389, f=w387) -> (s? t:f=w385:i32)
                            n171 = Build Array(w391, w385, u32 0 ("element")) -> (w392:u32[])
                            n172 = call-poly <vilib>:"Write To Spreadsheet File.vi"("append to file? (new file:F)"=TRUE, "1D data"=w392, "file path (dialog if empty)"=w393) -> ()  [unwired: 5 in, 1 out]
                          }
                          frame #2 {
                            w402 = u32 0 ("element")
                            n173 = call "3D_to_Pixels.vi"("Distance_3D"=w401) -> ("Distance_pixels"=w400:dbl)  [unwired: 11 in, 3 out]
                            n174 = Decrement(x=w403) -> (x-1=w396:u32)
                            n175 = Greater?(x=w396, y=u32 10000 ("element")) -> (0:w399:bool)
                            n176 = Select(t=1, s=w399, f=w396) -> (s? t:f=w395:u32)
                            n177 = Build Array(w400, w395, w402) -> (w406:dbl[])
                            n178 = call-poly <vilib>:"Write To Spreadsheet File.vi"("append to file? (new file:F)"=TRUE, "1D data"=w406, "file path (dialog if empty)"=w404) -> ()  [unwired: 5 in, 1 out]
                          }
                          frame #3 {
                            n179 = call "3D_to_Pixels.vi"("X_3D"=-0.8 ("element"), "Y_3D"=-0.8 ("element"), "Z_3D"=0.8 ("element")) -> ("X_pixels"=w411:dbl, "Y_pixels"=w412:dbl, "Z_pixels"=w413:dbl)  [unwired: 9 in, 1 out]
                            n180 = Build Array(w411, w412, w413) -> (w410:dbl[])
                            n181 = call-poly <vilib>:"Write To Spreadsheet File.vi"("append to file? (new file:F)"=TRUE, "1D data"=w410, "file path (dialog if empty)"=w414) -> ()  [unwired: 5 in, 1 out]
                          }
                          frame #4 {
                            n182 = call "3D_to_Pixels.vi"("X_3D"=0.8 ("element"), "Y_3D"=0.8 ("element"), "Z_3D"=-0.8 ("element")) -> ("X_pixels"=w420:dbl, "Y_pixels"=w421:dbl, "Z_pixels"=w422:dbl)  [unwired: 9 in, 1 out]
                            n183 = Build Array(w420, w421, w422) -> (w419:dbl[])
                            n184 = call-poly <vilib>:"Write To Spreadsheet File.vi"("append to file? (new file:F)"=TRUE, "1D data"=w419, "file path (dialog if empty)"=w423) -> ()  [unwired: 5 in, 1 out]
                          }
                        }
                      }
                    }
                  }
                }
              }
              frame 1 {
                n185 = Unbundle(w433) -> ("X_3D"=w448:dbl, "Y_3D"=w447:dbl, "Z"=w446:dbl)
                n186 = call "3D_Session_Data.vi"("Session"=w432) -> ("Radius"=w431:sgl, "min"=w436:dbl, "max"=w435:dbl)  [unwired: 8 in]
                n187 = Less Or Equal?(x=w448, y=w435) -> (x <= y?=w444:bool)
                n188 = Greater Or Equal?(x=w448, y=w436) -> (x >= y?=w445:bool)
                n189 = Less Or Equal?(x=w446, y=w435) -> (x <= y?=w440:bool)
                n190 = Greater Or Equal?(x=w446, y=w436) -> (x >= y?=w441:bool)
                n191 = Negate(x=w435) -> (-x=w438:dbl)
                n192 = Negate(x=w436) -> (-x=w437:dbl)
                n193 = Greater Or Equal?(x=w447, y=w438) -> (x >= y?=w443:bool)
                n194 = Less Or Equal?(x=w447, y=w437) -> (x <= y?=w442:bool)
                n195 = Build Array(w445, w444, w443, w442, w441, w440) -> (w439:bool[])
                n196 = And Array Elements(Boolean array=w439) -> (logical AND=w434:bool)
                n197 = case shown="True" w434 {
                  tunnel: [T12[] [{"Red"=0.0, "Green"=0.0, "Blue"=0.545, "Alpha"=0.8}, {"Red"=0.0, "Green"=0.0, "Blue"=0.545, "Alpha"=0.8}, {"Red"=0.0, "Green"=0.0, "Blue"=0.545, "Alpha"=0.8}, {"Red"=0.0, "Green"=0.0, "Blue"=0.545, "Alpha"=0.8}, {"Red"=0.0, "Green"=0.0, "Blue"=0.545, "Alpha"=0.8}, {"Red"=0.0, "Green"=0.0, "Blue"=0.545, "Alpha"=0.8}, {"Red"=0.0, "Green"=0.0, "Blue"=0.545, "Alpha"=0.8}, {"Red"=0.0, "Green"=1.0, "Blue"=1.0, "Alpha"=0.8}] ("Array") w510] -> w465
                  tunnel: [T11 {"Red"=1.0, "Green"=0.0, "Blue"=0.0, "Alpha"=1.0} ("Color") w509] -> w464
                  tunnel: w452 -> [w469 w508]
                  tunnel: w463 -> [w478 w507]
                  tunnel: [w478 w506] -> w462
                  tunnel: w461 -> [w477 w505]
                  tunnel: [w477 w504] -> w460
                  tunnel: w459 -> [_ w503]
                  tunnel: w431 -> [_ w502]
                  tunnel: [w476 w501] -> w458
                  tunnel: w457 -> [w476 w500]
                  tunnel: w456 -> [w473 w497]
                  tunnel: w455 -> [w472 w499]
                  tunnel: [w471 w497] -> w454
                  tunnel: [w470 w498] -> w453
                  tunnel: w433 -> [w468 w496]
                  tunnel: [w468 w495] -> w451
                  tunnel: [w467 w494] -> w450
                  tunnel: w449 -> [w467 w493]
                  frame False {
                    n198 = case shown="False" w469 {
                      tunnel: w473 -> [w480 w492]
                      tunnel: [w481 w491] -> w471
                      tunnel: w472 -> [w483 w490]
                      tunnel: [w482 w490] -> w470
                      frame False {
                        n199 = Greater Than 0?(x=w480) -> (x > 0?=w484:bool)
                        n200 = case shown="False" w484 {
                          tunnel: w483 -> [w486 w489]
                          tunnel: [w486 w488] -> w482
                          tunnel: w480 -> [w485 _]
                          tunnel: [w485 0 ("missed hits")] -> w481
                          frame False {
                          }
                          frame True {
                            n201 = Increment(x=w489) -> (x+1=w488:i32)
                          }
                        }
                      }
                      frame True {
                        n202 = Increment(x=w492) -> (x+1=w491:i32)
                      }
                    }
                    n203 = Number To Decimal String(number=0) -> (decimal integer string=w475:string)  [unwired: 1 in]
                    n204 = property on="initial time 2" class="DigNum (strict)"("NumText.Text"=w475) -> ()  [unwired: 2 in, 2 out]
                  }
                  frame True {
                    n205 = case shown="True" w508 {
                      tunnel: [T12[] [{"Red"=0.0, "Green"=0.0, "Blue"=0.545, "Alpha"=0.8}, {"Red"=0.0, "Green"=0.0, "Blue"=0.545, "Alpha"=0.8}, {"Red"=0.0, "Green"=0.0, "Blue"=0.545, "Alpha"=0.8}, {"Red"=0.0, "Green"=0.0, "Blue"=0.545, "Alpha"=0.8}, {"Red"=0.0, "Green"=0.0, "Blue"=0.545, "Alpha"=0.8}, {"Red"=0.0, "Green"=0.0, "Blue"=0.545, "Alpha"=0.8}, {"Red"=0.0, "Green"=0.0, "Blue"=0.545, "Alpha"=0.8}, {"Red"=0.0, "Green"=0.8, "Blue"=0.0, "Alpha"=0.8}] ("Array") T12[] [{"Red"=0.0, "Green"=0.0, "Blue"=0.545, "Alpha"=0.8}, {"Red"=0.0, "Green"=0.0, "Blue"=0.545, "Alpha"=0.8}, {"Red"=0.0, "Green"=0.0, "Blue"=0.545, "Alpha"=0.8}, {"Red"=0.0, "Green"=0.0, "Blue"=0.545, "Alpha"=0.8}, {"Red"=0.0, "Green"=0.0, "Blue"=0.545, "Alpha"=0.8}, {"Red"=0.0, "Green"=0.0, "Blue"=0.545, "Alpha"=0.8}, {"Red"=0.0, "Green"=0.0, "Blue"=0.545, "Alpha"=0.8}, {"Red"=1.0, "Green"=1.0, "Blue"=0.0, "Alpha"=0.8}] ("Array")] -> w510
                      tunnel: [T11 {"Red"=0.0, "Green"=0.8, "Blue"=0.0, "Alpha"=1.0} ("Color") T11 {"Red"=1.0, "Green"=1.0, "Blue"=0.0, "Alpha"=1.0} ("Color")] -> w509
                      tunnel: w507 -> [w521 w550]
                      tunnel: [w521 w549] -> w506
                      tunnel: w505 -> [w520 w533]
                      tunnel: [w520 w548] -> w504
                      tunnel: w503 -> [_ w543]
                      tunnel: w502 -> [_ w541]
                      tunnel: [w516 w540] -> w501
                      tunnel: w500 -> [w515 w539]
                      tunnel: w499 -> [w514 w532]
                      tunnel: [w514 0 ("x")] -> w498
                      tunnel: w496 -> [w513 _]
                      tunnel: [w513 w531] -> w495
                      tunnel: [w512 w530] -> w494
                      tunnel: w493 -> [w512 w529]
                      frame False {
                        n206 = property on="initial time 2" class="DigNum (strict)"() -> ("NumText.Text"=w518:string)  [unwired: 2 in, 2 out]
                        n207 = Decimal String To Number(string=w518) -> (number=w517:i32)  [unwired: 2 in, 1 out]
                        n208 = Equal To 0?(x=w517) -> (x = 0?=w519:bool)
                        n209 = case shown="False" w519 {
                          tunnel: w515 -> [w523 w527]
                          tunnel: [w523 w526] -> w516
                          frame False {
                          }
                          frame True {
                            n210 = Increment(x=w527) -> (x+1=w526:u32)
                            n211 = Number To Decimal String(number=1) -> (decimal integer string=w525:string)  [unwired: 1 in]
                            n212 = property on="initial time 2" class="DigNum (strict)"("NumText.Text"=w525) -> ()  [unwired: 2 in, 2 out]
                          }
                        }
                      }
                      frame True {
                        w531 = cluster{dbl, dbl, "y":dbl} {0.8, -0.8, "y"=-0.8}
                        n213 = stacked-sequence {
                          seq-local: [w597 _] -> [_ w600]
                          tunnel: [w596 _] -> w542
                          frame #0 {
                            n214 = property on="initial time" class="DigNum (strict)"() -> ("NumText.Text"=w599:string)  [unwired: 2 in, 2 out]
                            n215 = Decimal String To Number(string=w599) -> (number=w598:i32)  [unwired: 2 in, 1 out]
                            n216 = Tick Count (ms)() -> (millisecond timer value=w597:u32)
                            n217 = Subtract(x=w597, y=w598) -> (x-y=w596:u32)
                          }
                          frame #1 {
                            n218 = Number To Decimal String(number=w600) -> (decimal integer string=w601:string)  [unwired: 1 in]
                            n219 = property on="initial time" class="DigNum (strict)"("NumText.Text"=w601) -> ()  [unwired: 2 in, 2 out]
                          }
                        }
                        n220 = Increment(x=w533) -> (x+1=w548:i32)
                        n221 = Increment(x=w550) -> (x+1=w549:i32)
                        n222 = Current VI's Path() -> (path=w546:path)
                        n223 = Unbundle(w531) -> (w537:dbl, w538:dbl)  [unwired: 1 out]
                        n224 = Strip Path(path=w546) -> (stripped path=w545:path)  [unwired: 1 out]
                        n225 = call "3D_to_Screen.vi"("X_3D"=w537, "Y_3D"=w538) -> ("X"=w536:dbl, "Y"=w535:dbl)  [unwired: 11 in, 1 out]
                        n226 = dll-call lib="User32.dll" fn="SetCursorPos"(w536, w535) -> ()  [unwired: 6 in, 2 out]
                        n227 = Build Path(base path=w545, name or relative path="successful_hit.wav") -> (appended path=w547:path)
                        n228 = call <vilib>:"Play Sound File.vi"("path"=w547) -> ()  [unwired: 9 in, 2 out]
                        n229 = stacked-sequence {
                          tunnel: w543 -> [w552 w564 w575 w585 w594]
                          tunnel: w542 -> [_ w562 _ _ _]
                          tunnel: w541 -> [_ _ w572 _ _]
                          tunnel: [_ _ w573 _ _] -> w540
                          tunnel: w539 -> [_ _ w574 _ _]
                          tunnel: w532 -> [_ w557 _ _ _]
                          tunnel: [dbl[][] [] _ _ _ _] -> w530
                          tunnel: w529 -> [w554 _ _ _ _]
                          frame #0 {
                            n230 = call-poly <vilib>:"Write To Spreadsheet File.vi"("append to file? (new file:F)"=TRUE, "2D data"=w554, "file path (dialog if empty)"=w552) -> ()  [unwired: 5 in, 1 out]
                          }
                          frame #1 {
                            n231 = Greater?(x=w557, y=u32 10000 ("element")) -> (0:w560:bool)
                            n232 = Select(t=1, s=w560, f=w557) -> (s? t:f=w556:i32)
                            n233 = Build Array(w562, w556, u32 0 ("element")) -> (w563:u32[])
                            n234 = call-poly <vilib>:"Write To Spreadsheet File.vi"("append to file? (new file:F)"=TRUE, "1D data"=w563, "file path (dialog if empty)"=w564) -> ()  [unwired: 5 in, 1 out]
                          }
                          frame #2 {
                            w573 = u32 0 ("element")
                            n235 = call "3D_to_Pixels.vi"("Distance_3D"=w572) -> ("Distance_pixels"=w571:dbl)  [unwired: 11 in, 3 out]
                            n236 = Decrement(x=w574) -> (x-1=w567:u32)
                            n237 = Greater?(x=w567, y=u32 10000 ("element")) -> (0:w570:bool)
                            n238 = Select(t=1, s=w570, f=w567) -> (s? t:f=w566:u32)
                            n239 = Build Array(w571, w566, w573) -> (w577:dbl[])
                            n240 = call-poly <vilib>:"Write To Spreadsheet File.vi"("append to file? (new file:F)"=TRUE, "1D data"=w577, "file path (dialog if empty)"=w575) -> ()  [unwired: 5 in, 1 out]
                          }
                          frame #3 {
                            n241 = call "3D_to_Pixels.vi"("X_3D"=-0.8 ("element"), "Y_3D"=0.8 ("element"), "Z_3D"=-0.8 ("element")) -> ("X_pixels"=w582:dbl, "Y_pixels"=w583:dbl, "Z_pixels"=w584:dbl)  [unwired: 9 in, 1 out]
                            n242 = Build Array(w582, w583, w584) -> (w581:dbl[])
                            n243 = call-poly <vilib>:"Write To Spreadsheet File.vi"("append to file? (new file:F)"=TRUE, "1D data"=w581, "file path (dialog if empty)"=w585) -> ()  [unwired: 5 in, 1 out]
                          }
                          frame #4 {
                            n244 = call "3D_to_Pixels.vi"("X_3D"=0.8 ("element"), "Y_3D"=-0.8 ("element"), "Z_3D"=0.8 ("element")) -> ("X_pixels"=w593:dbl, "Y_pixels"=w592:dbl, "Z_pixels"=w591:dbl)  [unwired: 9 in, 1 out]
                            n245 = Build Array(w593, w592, w591) -> (w590:dbl[])
                            n246 = call-poly <vilib>:"Write To Spreadsheet File.vi"("append to file? (new file:F)"=TRUE, "1D data"=w590, "file path (dialog if empty)"=w594) -> ()  [unwired: 5 in, 1 out]
                          }
                        }
                      }
                    }
                  }
                }
              }
              frame 2 {
                n247 = Unbundle(w604) -> ("X_3D"=w619:dbl, "Y_3D"=w618:dbl, "Z"=w617:dbl)
                n248 = call "3D_Session_Data.vi"("Session"=w603) -> ("Radius"=w602:sgl, "min"=w607:dbl, "max"=w606:dbl)  [unwired: 8 in]
                n249 = Less Or Equal?(x=w618, y=w606) -> (x <= y?=w613:bool)
                n250 = Greater Or Equal?(x=w618, y=w607) -> (x >= y?=w614:bool)
                n251 = Less Or Equal?(x=w617, y=w606) -> (x <= y?=w611:bool)
                n252 = Greater Or Equal?(x=w617, y=w607) -> (x >= y?=w612:bool)
                n253 = Negate(x=w606) -> (-x=w609:dbl)
                n254 = Negate(x=w607) -> (-x=w608:dbl)
                n255 = Greater Or Equal?(x=w619, y=w609) -> (x >= y?=w616:bool)
                n256 = Less Or Equal?(x=w619, y=w608) -> (x <= y?=w615:bool)
                n257 = Build Array(w616, w615, w614, w613, w612, w611) -> (w610:bool[])
                n258 = And Array Elements(Boolean array=w610) -> (logical AND=w605:bool)
                n259 = case shown="True" w605 {
                  tunnel: [T12[] [{"Red"=0.0, "Green"=0.0, "Blue"=0.545, "Alpha"=0.8}, {"Red"=0.0, "Green"=0.0, "Blue"=0.545, "Alpha"=0.8}, {"Red"=0.0, "Green"=0.0, "Blue"=0.545, "Alpha"=0.8}, {"Red"=0.0, "Green"=0.0, "Blue"=0.545, "Alpha"=0.8}, {"Red"=0.0, "Green"=1.0, "Blue"=1.0, "Alpha"=0.8}, {"Red"=0.0, "Green"=0.0, "Blue"=0.545, "Alpha"=0.8}, {"Red"=0.0, "Green"=0.0, "Blue"=0.545, "Alpha"=0.8}, {"Red"=0.0, "Green"=0.0, "Blue"=0.545, "Alpha"=0.8}] ("Array") w681] -> w636
                  tunnel: [T11 {"Red"=1.0, "Green"=0.0, "Blue"=0.0, "Alpha"=1.0} ("Color") w680] -> w635
                  tunnel: w634 -> [w640 w679]
                  tunnel: w633 -> [w649 w678]
                  tunnel: [w649 w677] -> w632
                  tunnel: w631 -> [w648 w676]
                  tunnel: [w648 w675] -> w630
                  tunnel: w629 -> [_ w674]
                  tunnel: w602 -> [_ w673]
                  tunnel: [w647 w672] -> w628
                  tunnel: w627 -> [w647 w671]
                  tunnel: w626 -> [w644 w668]
                  tunnel: w625 -> [w643 w670]
                  tunnel: [w642 w668] -> w624
                  tunnel: [w641 w669] -> w623
                  tunnel: w604 -> [w639 w667]
                  tunnel: [w639 w666] -> w622
                  tunnel: w621 -> [w638 w665]
                  tunnel: [w638 w664] -> w620
                  frame False {
                    n260 = case shown="True" w640 {
                      tunnel: w644 -> [w651 w663]
                      tunnel: [w652 w662] -> w642
                      tunnel: w643 -> [w654 w661]
                      tunnel: [w653 w661] -> w641
                      frame False {
                        n261 = Greater Than 0?(x=w651) -> (x > 0?=w655:bool)
                        n262 = case shown="False" w655 {
                          tunnel: w654 -> [w657 w660]
                          tunnel: [w657 w659] -> w653
                          tunnel: w651 -> [w656 _]
                          tunnel: [w656 0 ("y")] -> w652
                          frame False {
                          }
                          frame True {
                            n263 = Increment(x=w660) -> (x+1=w659:i32)
                          }
                        }
                      }
                      frame True {
                        n264 = Increment(x=w663) -> (x+1=w662:i32)
                      }
                    }
                    n265 = Number To Decimal String(number=0) -> (decimal integer string=w646:string)  [unwired: 1 in]
                    n266 = property on="initial time 2" class="DigNum (strict)"("NumText.Text"=w646) -> ()  [unwired: 2 in, 2 out]
                  }
                  frame True {
                    n267 = case shown="True" w679 {
                      tunnel: [T12[] [{"Red"=0.0, "Green"=0.0, "Blue"=0.545, "Alpha"=0.8}, {"Red"=0.0, "Green"=0.0, "Blue"=0.545, "Alpha"=0.8}, {"Red"=0.0, "Green"=0.0, "Blue"=0.545, "Alpha"=0.8}, {"Red"=0.0, "Green"=0.0, "Blue"=0.545, "Alpha"=0.8}, {"Red"=0.0, "Green"=0.8, "Blue"=0.0, "Alpha"=0.8}, {"Red"=0.0, "Green"=0.0, "Blue"=0.545, "Alpha"=0.8}, {"Red"=0.0, "Green"=0.0, "Blue"=0.545, "Alpha"=0.8}, {"Red"=0.0, "Green"=0.0, "Blue"=0.545, "Alpha"=0.8}] ("Array") T12[] [{"Red"=0.0, "Green"=0.0, "Blue"=0.545, "Alpha"=0.8}, {"Red"=0.0, "Green"=0.0, "Blue"=0.545, "Alpha"=0.8}, {"Red"=0.0, "Green"=0.0, "Blue"=0.545, "Alpha"=0.8}, {"Red"=0.0, "Green"=0.0, "Blue"=0.545, "Alpha"=0.8}, {"Red"=1.0, "Green"=1.0, "Blue"=0.0, "Alpha"=0.8}, {"Red"=0.0, "Green"=0.0, "Blue"=0.545, "Alpha"=0.8}, {"Red"=0.0, "Green"=0.0, "Blue"=0.545, "Alpha"=0.8}, {"Red"=0.0, "Green"=0.0, "Blue"=0.545, "Alpha"=0.8}] ("Array")] -> w681
                      tunnel: [T11 {"Red"=0.0, "Green"=0.8, "Blue"=0.0, "Alpha"=1.0} ("Color") T11 {"Red"=1.0, "Green"=1.0, "Blue"=0.0, "Alpha"=1.0} ("Color")] -> w680
                      tunnel: w678 -> [w692 w721]
                      tunnel: [w692 w720] -> w677
                      tunnel: w676 -> [w691 w719]
                      tunnel: [w691 w718] -> w675
                      tunnel: w674 -> [_ w712]
                      tunnel: w673 -> [_ w711]
                      tunnel: [w686 w710] -> w672
                      tunnel: w671 -> [w687 w709]
                      tunnel: w670 -> [w685 w708]
                      tunnel: [w685 0 ("missed clicks")] -> w669
                      tunnel: w667 -> [w684 _]
                      tunnel: [w684 w702] -> w666
                      tunnel: w665 -> [w683 w701]
                      tunnel: [w683 w700] -> w664
                      frame False {
                        n268 = property on="initial time 2" class="DigNum (strict)"() -> ("NumText.Text"=w689:string)  [unwired: 2 in, 2 out]
                        n269 = Decimal String To Number(string=w689) -> (number=w688:i32)  [unwired: 2 in, 1 out]
                        n270 = Equal To 0?(x=w688) -> (x = 0?=w690:bool)
                        n271 = case shown="True" w690 {
                          tunnel: w687 -> [w694 w698]
                          tunnel: [w694 w697] -> w686
                          frame False {
                          }
                          frame True {
                            n272 = Increment(x=w698) -> (x+1=w697:u32)
                            n273 = Number To Decimal String(number=1) -> (decimal integer string=w696:string)  [unwired: 1 in]
                            n274 = property on="initial time 2" class="DigNum (strict)"("NumText.Text"=w696) -> ()  [unwired: 2 in, 2 out]
                          }
                        }
                      }
                      frame True {
                        w702 = cluster{dbl, dbl, "y":dbl} {0.8, 0.8, "y"=0.8}
                        n275 = stacked-sequence {
                          seq-local: [w768 _] -> [_ w771]
                          tunnel: [w767 _] -> w713
                          frame #0 {
                            n276 = property on="initial time" class="DigNum (strict)"() -> ("NumText.Text"=w770:string)  [unwired: 2 in, 2 out]
                            n277 = Decimal String To Number(string=w770) -> (number=w769:i32)  [unwired: 2 in, 1 out]
                            n278 = Tick Count (ms)() -> (millisecond timer value=w768:u32)
                            n279 = Subtract(x=w768, y=w769) -> (x-y=w767:u32)
                          }
                          frame #1 {
                            n280 = Number To Decimal String(number=w771) -> (decimal integer string=w772:string)  [unwired: 1 in]
                            n281 = property on="initial time" class="DigNum (strict)"("NumText.Text"=w772) -> ()  [unwired: 2 in, 2 out]
                          }
                        }
                        n282 = Increment(x=w719) -> (x+1=w718:i32)
                        n283 = Increment(x=w721) -> (x+1=w720:i32)
                        n284 = Current VI's Path() -> (path=w716:path)
                        n285 = Unbundle(w702) -> (w707:dbl, w706:dbl)  [unwired: 1 out]
                        n286 = Strip Path(path=w716) -> (stripped path=w715:path)  [unwired: 1 out]
                        n287 = call "3D_to_Screen.vi"("X_3D"=w707, "Y_3D"=w706) -> ("X"=w705:dbl, "Y"=w704:dbl)  [unwired: 11 in, 1 out]
                        n288 = dll-call lib="User32.dll" fn="SetCursorPos"(w705, w704) -> ()  [unwired: 6 in, 2 out]
                        n289 = Build Path(base path=w715, name or relative path="successful_hit.wav") -> (appended path=w717:path)
                        n290 = call <vilib>:"Play Sound File.vi"("path"=w717) -> ()  [unwired: 9 in, 2 out]
                        n291 = stacked-sequence {
                          tunnel: w712 -> [w723 w735 w746 w756 w765]
                          tunnel: w713 -> [_ w733 _ _ _]
                          tunnel: w711 -> [_ _ w742 _ _]
                          tunnel: [_ _ w744 _ _] -> w710
                          tunnel: w709 -> [_ _ w745 _ _]
                          tunnel: w708 -> [_ w728 _ _ _]
                          tunnel: w701 -> [w725 _ _ _ _]
                          tunnel: [dbl[][] [] _ _ _ _] -> w700
                          frame #0 {
                            n292 = call-poly <vilib>:"Write To Spreadsheet File.vi"("append to file? (new file:F)"=TRUE, "2D data"=w725, "file path (dialog if empty)"=w723) -> ()  [unwired: 5 in, 1 out]
                          }
                          frame #1 {
                            n293 = Greater?(x=w728, y=u32 10000 ("element")) -> (0:w731:bool)
                            n294 = Select(t=1, s=w731, f=w728) -> (s? t:f=w727:i32)
                            n295 = Build Array(w733, w727, u32 0 ("element")) -> (w734:u32[])
                            n296 = call-poly <vilib>:"Write To Spreadsheet File.vi"("append to file? (new file:F)"=TRUE, "1D data"=w734, "file path (dialog if empty)"=w735) -> ()  [unwired: 5 in, 1 out]
                          }
                          frame #2 {
                            w744 = u32 0 ("element")
                            n297 = call "3D_to_Pixels.vi"("Distance_3D"=w742) -> ("Distance_pixels"=w743:dbl)  [unwired: 11 in, 3 out]
                            n298 = Decrement(x=w745) -> (x-1=w738:u32)
                            n299 = Greater?(x=w738, y=u32 10000 ("element")) -> (0:w741:bool)
                            n300 = Select(t=1, s=w741, f=w738) -> (s? t:f=w737:u32)
                            n301 = Build Array(w743, w737, w744) -> (w747:dbl[])
                            n302 = call-poly <vilib>:"Write To Spreadsheet File.vi"("append to file? (new file:F)"=TRUE, "1D data"=w747, "file path (dialog if empty)"=w746) -> ()  [unwired: 5 in, 1 out]
                          }
                          frame #3 {
                            n303 = call "3D_to_Pixels.vi"("X_3D"=0.8 ("element"), "Y_3D"=-0.8 ("element"), "Z_3D"=-0.8 ("element")) -> ("X_pixels"=w755:dbl, "Y_pixels"=w754:dbl, "Z_pixels"=w753:dbl)  [unwired: 9 in, 1 out]
                            n304 = Build Array(w755, w754, w753) -> (w752:dbl[])
                            n305 = call-poly <vilib>:"Write To Spreadsheet File.vi"("append to file? (new file:F)"=TRUE, "1D data"=w752, "file path (dialog if empty)"=w756) -> ()  [unwired: 5 in, 1 out]
                          }
                          frame #4 {
                            n306 = call "3D_to_Pixels.vi"("X_3D"=-0.8 ("element"), "Y_3D"=0.8 ("element"), "Z_3D"=0.8 ("element")) -> ("X_pixels"=w764:dbl, "Y_pixels"=w763:dbl, "Z_pixels"=w762:dbl)  [unwired: 9 in, 1 out]
                            n307 = Build Array(w764, w763, w762) -> (w761:dbl[])
                            n308 = call-poly <vilib>:"Write To Spreadsheet File.vi"("append to file? (new file:F)"=TRUE, "1D data"=w761, "file path (dialog if empty)"=w765) -> ()  [unwired: 5 in, 1 out]
                          }
                        }
                      }
                    }
                  }
                }
              }
              frame 3 {
                n309 = call "3D_Session_Data.vi"("Session"=w773) -> ("Radius"=w776:sgl, "min"=w780:dbl, "max"=w774:dbl)  [unwired: 8 in]
                n310 = Unbundle(w775) -> ("X_3D"=w790:dbl, "Y_3D"=w789:dbl, "Z"=w788:dbl)
                n311 = Negate(x=w774) -> (-x=w779:dbl)
                n312 = Negate(x=w780) -> (-x=w778:dbl)
                n313 = Greater Or Equal?(x=w790, y=w779) -> (x >= y?=w787:bool)
                n314 = Greater Or Equal?(x=w789, y=w779) -> (x >= y?=w785:bool)
                n315 = Greater Or Equal?(x=w788, y=w779) -> (x >= y?=w783:bool)
                n316 = Less Or Equal?(x=w790, y=w778) -> (x <= y?=w786:bool)
                n317 = Less Or Equal?(x=w789, y=w778) -> (x <= y?=w784:bool)
                n318 = Less Or Equal?(x=w788, y=w778) -> (x <= y?=w782:bool)
                n319 = Build Array(w787, w786, w785, w784, w783, w782) -> (w781:bool[])
                n320 = And Array Elements(Boolean array=w781) -> (logical AND=w777:bool)
                n321 = case shown="True" w777 {
                  tunnel: [T12[] [{"Red"=0.0, "Green"=0.0, "Blue"=0.545, "Alpha"=0.8}, {"Red"=0.0, "Green"=0.0, "Blue"=0.545, "Alpha"=0.8}, {"Red"=0.0, "Green"=0.0, "Blue"=0.545, "Alpha"=0.8}, {"Red"=0.0, "Green"=1.0, "Blue"=1.0, "Alpha"=0.8}, {"Red"=0.0, "Green"=0.0, "Blue"=0.545, "Alpha"=0.8}, {"Red"=0.0, "Green"=0.0, "Blue"=0.545, "Alpha"=0.8}, {"Red"=0.0, "Green"=0.0, "Blue"=0.545, "Alpha"=0.8}, {"Red"=0.0, "Green"=0.0, "Blue"=0.545, "Alpha"=0.8}] ("Array") w852] -> w807
                  tunnel: [T11 {"Red"=1.0, "Green"=0.0, "Blue"=0.0, "Alpha"=1.0} ("Color") w851] -> w806
                  tunnel: w805 -> [w811 w850]
                  tunnel: w804 -> [w820 w849]
                  tunnel: [w820 w848] -> w803
                  tunnel: w802 -> [w819 w847]
                  tunnel: [w819 w846] -> w801
                  tunnel: w800 -> [_ w845]
                  tunnel: w776 -> [_ w844]
                  tunnel: [w818 w843] -> w799
                  tunnel: w798 -> [w818 w842]
                  tunnel: w797 -> [w815 w841]
                  tunnel: w796 -> [w814 w840]
                  tunnel: [w813 w841] -> w795
                  tunnel: [w812 w839] -> w794
                  tunnel: w775 -> [w810 w838]
                  tunnel: [w810 w837] -> w793
                  tunnel: w792 -> [w809 w836]
                  tunnel: [w809 w835] -> w791
                  frame False {
                    n322 = case shown="False" w811 {
                      tunnel: w815 -> [w823 w834]
                      tunnel: [w822 w833] -> w813
                      tunnel: w814 -> [w825 w832]
                      tunnel: [w824 w832] -> w812
                      frame False {
                        n323 = Equal To 0?(x=w823) -> (x = 0?=w826:bool)
                        n324 = case shown="True" w826 {
                          tunnel: w825 -> [w828 w831]
                          tunnel: [w828 w830] -> w824
                          tunnel: w823 -> [w827 _]
                          tunnel: [w827 0 ("y")] -> w822
                          frame False {
                          }
                          frame True {
                            n325 = Increment(x=w831) -> (x+1=w830:i32)
                          }
                        }
                      }
                      frame True {
                        n326 = Increment(x=w834) -> (x+1=w833:i32)
                      }
                    }
                    n327 = Number To Decimal String(number=0) -> (decimal integer string=w817:string)  [unwired: 1 in]
                    n328 = property on="initial time 2" class="DigNum (strict)"("NumText.Text"=w817) -> ()  [unwired: 2 in, 2 out]
                  }
                  frame True {
                    n329 = case shown="True" w850 {
                      tunnel: [T12[] [{"Red"=0.0, "Green"=0.0, "Blue"=0.545, "Alpha"=0.8}, {"Red"=0.0, "Green"=0.0, "Blue"=0.545, "Alpha"=0.8}, {"Red"=0.0, "Green"=0.0, "Blue"=0.545, "Alpha"=0.8}, {"Red"=0.0, "Green"=0.8, "Blue"=0.0, "Alpha"=0.8}, {"Red"=0.0, "Green"=0.0, "Blue"=0.545, "Alpha"=0.8}, {"Red"=0.0, "Green"=0.0, "Blue"=0.545, "Alpha"=0.8}, {"Red"=0.0, "Green"=0.0, "Blue"=0.545, "Alpha"=0.8}, {"Red"=0.0, "Green"=0.0, "Blue"=0.545, "Alpha"=0.8}] ("Array") T12[] [{"Red"=0.0, "Green"=0.0, "Blue"=0.545, "Alpha"=0.8}, {"Red"=0.0, "Green"=0.0, "Blue"=0.545, "Alpha"=0.8}, {"Red"=0.0, "Green"=0.0, "Blue"=0.545, "Alpha"=0.8}, {"Red"=1.0, "Green"=1.0, "Blue"=0.0, "Alpha"=0.8}, {"Red"=0.0, "Green"=0.0, "Blue"=0.545, "Alpha"=0.8}, {"Red"=0.0, "Green"=0.0, "Blue"=0.545, "Alpha"=0.8}, {"Red"=0.0, "Green"=0.0, "Blue"=0.545, "Alpha"=0.8}, {"Red"=0.0, "Green"=0.0, "Blue"=0.545, "Alpha"=0.8}] ("Array")] -> w852
                      tunnel: [T11 {"Red"=0.0, "Green"=0.8, "Blue"=0.0, "Alpha"=1.0} ("Color") T11 {"Red"=1.0, "Green"=1.0, "Blue"=0.0, "Alpha"=1.0} ("Color")] -> w851
                      tunnel: w849 -> [w863 w892]
                      tunnel: [w863 w891] -> w848
                      tunnel: w847 -> [w862 w890]
                      tunnel: [w862 w889] -> w846
                      tunnel: w845 -> [_ w883]
                      tunnel: w844 -> [_ w882]
                      tunnel: [w857 w881] -> w843
                      tunnel: w842 -> [w858 w880]
                      tunnel: w840 -> [w856 w879]
                      tunnel: [w856 0 ("y")] -> w839
                      tunnel: w838 -> [w855 _]
                      tunnel: [w855 w873] -> w837
                      tunnel: w836 -> [w854 w872]
                      tunnel: [w854 w871] -> w835
                      frame False {
                        n330 = property on="initial time 2" class="DigNum (strict)"() -> ("NumText.Text"=w860:string)  [unwired: 2 in, 2 out]
                        n331 = Decimal String To Number(string=w860) -> (number=w859:i32)  [unwired: 2 in, 1 out]
                        n332 = Equal To 0?(x=w859) -> (x = 0?=w861:bool)
                        n333 = case shown="False" w861 {
                          tunnel: w858 -> [w865 w869]
                          tunnel: [w865 w868] -> w857
                          frame False {
                          }
                          frame True {
                            n334 = Increment(x=w869) -> (x+1=w868:u32)
                            n335 = Number To Decimal String(number=1) -> (decimal integer string=w867:string)  [unwired: 1 in]
                            n336 = property on="initial time 2" class="DigNum (strict)"("NumText.Text"=w867) -> ()  [unwired: 2 in, 2 out]
                          }
                        }
                      }
                      frame True {
                        w873 = cluster{dbl, dbl, "y":dbl} {-0.8, -0.8, "y"=-0.8}
                        n337 = stacked-sequence {
                          seq-local: [w939 _] -> [_ w942]
                          tunnel: [w938 _] -> w884
                          frame #0 {
                            n338 = property on="initial time" class="DigNum (strict)"() -> ("NumText.Text"=w941:string)  [unwired: 2 in, 2 out]
                            n339 = Decimal String To Number(string=w941) -> (number=w940:i32)  [unwired: 2 in, 1 out]
                            n340 = Tick Count (ms)() -> (millisecond timer value=w939:u32)
                            n341 = Subtract(x=w939, y=w940) -> (x-y=w938:u32)
                          }
                          frame #1 {
                            n342 = Number To Decimal String(number=w942) -> (decimal integer string=w943:string)  [unwired: 1 in]
                            n343 = property on="initial time" class="DigNum (strict)"("NumText.Text"=w943) -> ()  [unwired: 2 in, 2 out]
                          }
                        }
                        n344 = Increment(x=w890) -> (x+1=w889:i32)
                        n345 = Increment(x=w892) -> (x+1=w891:i32)
                        n346 = Current VI's Path() -> (path=w887:path)
                        n347 = Unbundle(w873) -> (w878:dbl, w877:dbl)  [unwired: 1 out]
                        n348 = Strip Path(path=w887) -> (stripped path=w886:path)  [unwired: 1 out]
                        n349 = call "3D_to_Screen.vi"("X_3D"=w878, "Y_3D"=w877) -> ("X"=w876:dbl, "Y"=w875:dbl)  [unwired: 11 in, 1 out]
                        n350 = dll-call lib="User32.dll" fn="SetCursorPos"(w876, w875) -> ()  [unwired: 6 in, 2 out]
                        n351 = Build Path(base path=w886, name or relative path="successful_hit.wav") -> (appended path=w888:path)
                        n352 = call <vilib>:"Play Sound File.vi"("path"=w888) -> ()  [unwired: 9 in, 2 out]
                        n353 = stacked-sequence {
                          tunnel: w883 -> [w894 w906 w917 w927 w936]
                          tunnel: w884 -> [_ w904 _ _ _]
                          tunnel: w882 -> [_ _ w914 _ _]
                          tunnel: [_ _ w915 _ _] -> w881
                          tunnel: w880 -> [_ _ w916 _ _]
                          tunnel: w879 -> [_ w899 _ _ _]
                          tunnel: w872 -> [w895 _ _ _ _]
                          tunnel: [dbl[][] [] _ _ _ _] -> w871
                          frame #0 {
                            n354 = call-poly <vilib>:"Write To Spreadsheet File.vi"("append to file? (new file:F)"=TRUE, "2D data"=w895, "file path (dialog if empty)"=w894) -> ()  [unwired: 5 in, 1 out]
                          }
                          frame #1 {
                            n355 = Greater?(x=w899, y=u32 10000 ("element")) -> (0:w902:bool)
                            n356 = Select(t=1, s=w902, f=w899) -> (s? t:f=w898:i32)
                            n357 = Build Array(w904, w898, u32 0 ("element")) -> (w905:u32[])
                            n358 = call-poly <vilib>:"Write To Spreadsheet File.vi"("append to file? (new file:F)"=TRUE, "1D data"=w905, "file path (dialog if empty)"=w906) -> ()  [unwired: 5 in, 1 out]
                          }
                          frame #2 {
                            w915 = u32 0 ("element")
                            n359 = call "3D_to_Pixels.vi"("Distance_3D"=w914) -> ("Distance_pixels"=w913:dbl)  [unwired: 11 in, 3 out]
                            n360 = Decrement(x=w916) -> (x-1=w909:u32)
                            n361 = Greater?(x=w909, y=u32 10000 ("element")) -> (0:w912:bool)
                            n362 = Select(t=1, s=w912, f=w909) -> (s? t:f=w908:u32)
                            n363 = Build Array(w913, w908, w915) -> (w918:dbl[])
                            n364 = call-poly <vilib>:"Write To Spreadsheet File.vi"("append to file? (new file:F)"=TRUE, "1D data"=w918, "file path (dialog if empty)"=w917) -> ()  [unwired: 5 in, 1 out]
                          }
                          frame #3 {
                            n365 = call "3D_to_Pixels.vi"("X_3D"=0.8 ("element"), "Y_3D"=0.8 ("element"), "Z_3D"=0.8 ("element")) -> ("X_pixels"=w926:dbl, "Y_pixels"=w925:dbl, "Z_pixels"=w924:dbl)  [unwired: 9 in, 1 out]
                            n366 = Build Array(w926, w925, w924) -> (w923:dbl[])
                            n367 = call-poly <vilib>:"Write To Spreadsheet File.vi"("append to file? (new file:F)"=TRUE, "1D data"=w923, "file path (dialog if empty)"=w927) -> ()  [unwired: 5 in, 1 out]
                          }
                          frame #4 {
                            n368 = call "3D_to_Pixels.vi"("X_3D"=-0.8 ("element"), "Y_3D"=-0.8 ("element"), "Z_3D"=-0.8 ("element")) -> ("X_pixels"=w935:dbl, "Y_pixels"=w934:dbl, "Z_pixels"=w933:dbl)  [unwired: 9 in, 1 out]
                            n369 = Build Array(w935, w934, w933) -> (w929:dbl[])
                            n370 = call-poly <vilib>:"Write To Spreadsheet File.vi"("append to file? (new file:F)"=TRUE, "1D data"=w929, "file path (dialog if empty)"=w936) -> ()  [unwired: 5 in, 1 out]
                          }
                        }
                      }
                    }
                  }
                }
              }
              frame 4 {
                n371 = Unbundle(w945) -> ("X_3D"=w959:dbl, "Y_3D"=w958:dbl, "Z"=w957:dbl)
                n372 = call "3D_Session_Data.vi"("Session"=w946) -> ("Radius"=w944:sgl, "min"=w949:dbl, "max"=w948:dbl)  [unwired: 8 in]
                n373 = Less Or Equal?(x=w959, y=w948) -> (x <= y?=w955:bool)
                n374 = Greater Or Equal?(x=w959, y=w949) -> (x >= y?=w956:bool)
                n375 = Less Or Equal?(x=w958, y=w948) -> (x <= y?=w953:bool)
                n376 = Greater Or Equal?(x=w958, y=w949) -> (x >= y?=w954:bool)
                n377 = Less Or Equal?(x=w957, y=w948) -> (x <= y?=w951:bool)
                n378 = Greater Or Equal?(x=w957, y=w949) -> (x >= y?=w952:bool)
                n379 = Build Array(w956, w955, w954, w953, w952, w951) -> (w950:bool[])
                n380 = And Array Elements(Boolean array=w950) -> (logical AND=w947:bool)
                n381 = case shown="True" w947 {
                  tunnel: [T12[] [{"Red"=0.0, "Green"=0.0, "Blue"=0.545, "Alpha"=0.8}, {"Red"=0.0, "Green"=0.0, "Blue"=0.545, "Alpha"=0.8}, {"Red"=0.0, "Green"=1.0, "Blue"=1.0, "Alpha"=0.8}, {"Red"=0.0, "Green"=0.0, "Blue"=0.545, "Alpha"=0.8}, {"Red"=0.0, "Green"=0.0, "Blue"=0.545, "Alpha"=0.8}, {"Red"=0.0, "Green"=0.0, "Blue"=0.545, "Alpha"=0.8}, {"Red"=0.0, "Green"=0.0, "Blue"=0.545, "Alpha"=0.8}, {"Red"=0.0, "Green"=0.0, "Blue"=0.545, "Alpha"=0.8}] ("Array") w1021] -> w976
                  tunnel: [T11 {"Red"=1.0, "Green"=0.0, "Blue"=0.0, "Alpha"=1.0} ("Color") w1020] -> w975
                  tunnel: w974 -> [w980 w1019]
                  tunnel: w973 -> [w989 w1018]
                  tunnel: [w989 w1017] -> w972
                  tunnel: w971 -> [w988 w1016]
                  tunnel: [w988 w1015] -> w970
                  tunnel: w969 -> [_ w1014]
                  tunnel: w944 -> [_ w1013]
                  tunnel: [w987 w1011] -> w968
                  tunnel: w967 -> [w987 w1012]
                  tunnel: w966 -> [w984 w1010]
                  tunnel: w965 -> [w983 w1009]
                  tunnel: [w982 w1010] -> w964
                  tunnel: [w981 w1008] -> w963
                  tunnel: w945 -> [w979 w1007]
                  tunnel: [w979 w1006] -> w962
                  tunnel: w961 -> [w978 w1005]
                  tunnel: [w978 w1004] -> w960
                  frame False {
                    n382 = case shown="False" w980 {
                      tunnel: w984 -> [w992 w1003]
                      tunnel: [w991 w1002] -> w982
                      tunnel: w983 -> [w994 w1001]
                      tunnel: [w993 w1001] -> w981
                      frame False {
                        n383 = Greater Than 0?(x=w992) -> (x > 0?=w995:bool)
                        n384 = case shown="False" w995 {
                          tunnel: w994 -> [w997 w1000]
                          tunnel: [w997 w999] -> w993
                          tunnel: w992 -> [w996 _]
                          tunnel: [w996 0 ("y")] -> w991
                          frame False {
                          }
                          frame True {
                            n385 = Increment(x=w1000) -> (x+1=w999:i32)
                          }
                        }
                      }
                      frame True {
                        n386 = Increment(x=w1003) -> (x+1=w1002:i32)
                      }
                    }
                    n387 = Number To Decimal String(number=0) -> (decimal integer string=w986:string)  [unwired: 1 in]
                    n388 = property on="initial time 2" class="DigNum (strict)"("NumText.Text"=w986) -> ()  [unwired: 2 in, 2 out]
                  }
                  frame True {
                    n389 = case shown="True" w1019 {
                      tunnel: [T12[] [{"Red"=0.0, "Green"=0.0, "Blue"=0.545, "Alpha"=0.8}, {"Red"=0.0, "Green"=0.0, "Blue"=0.545, "Alpha"=0.8}, {"Red"=0.0, "Green"=0.8, "Blue"=0.0, "Alpha"=0.8}, {"Red"=0.0, "Green"=0.0, "Blue"=0.545, "Alpha"=0.8}, {"Red"=0.0, "Green"=0.0, "Blue"=0.545, "Alpha"=0.8}, {"Red"=0.0, "Green"=0.0, "Blue"=0.545, "Alpha"=0.8}, {"Red"=0.0, "Green"=0.0, "Blue"=0.545, "Alpha"=0.8}, {"Red"=0.0, "Green"=0.0, "Blue"=0.545, "Alpha"=0.8}] ("Array") T12[] [{"Red"=0.0, "Green"=0.0, "Blue"=0.545, "Alpha"=0.8}, {"Red"=0.0, "Green"=0.0, "Blue"=0.545, "Alpha"=0.8}, {"Red"=1.0, "Green"=1.0, "Blue"=0.0, "Alpha"=0.8}, {"Red"=0.0, "Green"=0.0, "Blue"=0.545, "Alpha"=0.8}, {"Red"=0.0, "Green"=0.0, "Blue"=0.545, "Alpha"=0.8}, {"Red"=0.0, "Green"=0.0, "Blue"=0.545, "Alpha"=0.8}, {"Red"=0.0, "Green"=0.0, "Blue"=0.545, "Alpha"=0.8}, {"Red"=0.0, "Green"=0.0, "Blue"=0.545, "Alpha"=0.8}] ("Array")] -> w1021
                      tunnel: [T11 {"Red"=0.0, "Green"=0.8, "Blue"=0.0, "Alpha"=1.0} ("Color") T11 {"Red"=1.0, "Green"=1.0, "Blue"=0.0, "Alpha"=1.0} ("Color")] -> w1020
                      tunnel: w1018 -> [w1032 w1061]
                      tunnel: [w1032 w1060] -> w1017
                      tunnel: w1016 -> [w1031 w1059]
                      tunnel: [w1031 w1058] -> w1015
                      tunnel: w1014 -> [_ w1052]
                      tunnel: w1013 -> [_ w1051]
                      tunnel: w1012 -> [w1027 w1049]
                      tunnel: [w1026 w1050] -> w1011
                      tunnel: w1009 -> [w1025 w1048]
                      tunnel: [w1025 0 ("y")] -> w1008
                      tunnel: w1007 -> [w1024 _]
                      tunnel: [w1024 w1042] -> w1006
                      tunnel: w1005 -> [w1023 w1041]
                      tunnel: [w1023 w1040] -> w1004
                      frame False {
                        n390 = property on="initial time 2" class="DigNum (strict)"() -> ("NumText.Text"=w1029:string)  [unwired: 2 in, 2 out]
                        n391 = Decimal String To Number(string=w1029) -> (number=w1028:i32)  [unwired: 2 in, 1 out]
                        n392 = Equal To 0?(x=w1028) -> (x = 0?=w1030:bool)
                        n393 = case shown="True" w1030 {
                          tunnel: w1027 -> [w1034 w1038]
                          tunnel: [w1034 w1037] -> w1026
                          frame False {
                          }
                          frame True {
                            n394 = Increment(x=w1038) -> (x+1=w1037:u32)
                            n395 = Number To Decimal String(number=1) -> (decimal integer string=w1036:string)  [unwired: 1 in]
                            n396 = property on="initial time 2" class="DigNum (strict)"("NumText.Text"=w1036) -> ()  [unwired: 2 in, 2 out]
                          }
                        }
                      }
                      frame True {
                        w1042 = cluster{dbl, dbl, "y":dbl} {-0.8, 0.8, "y"=0.8}
                        n397 = stacked-sequence {
                          seq-local: [w1108 _] -> [_ w1111]
                          tunnel: [w1107 _] -> w1053
                          frame #0 {
                            n398 = property on="initial time" class="DigNum (strict)"() -> ("NumText.Text"=w1110:string)  [unwired: 2 in, 2 out]
                            n399 = Decimal String To Number(string=w1110) -> (number=w1109:i32)  [unwired: 2 in, 1 out]
                            n400 = Tick Count (ms)() -> (millisecond timer value=w1108:u32)
                            n401 = Subtract(x=w1108, y=w1109) -> (x-y=w1107:u32)
                          }
                          frame #1 {
                            n402 = Number To Decimal String(number=w1111) -> (decimal integer string=w1112:string)  [unwired: 1 in]
                            n403 = property on="initial time" class="DigNum (strict)"("NumText.Text"=w1112) -> ()  [unwired: 2 in, 2 out]
                          }
                        }
                        n404 = Increment(x=w1059) -> (x+1=w1058:i32)
                        n405 = Increment(x=w1061) -> (x+1=w1060:i32)
                        n406 = Current VI's Path() -> (path=w1056:path)
                        n407 = Unbundle(w1042) -> (w1046:dbl, w1047:dbl)  [unwired: 1 out]
                        n408 = Strip Path(path=w1056) -> (stripped path=w1055:path)  [unwired: 1 out]
                        n409 = call "3D_to_Screen.vi"("X_3D"=w1046, "Y_3D"=w1047) -> ("X"=w1045:dbl, "Y"=w1044:dbl)  [unwired: 11 in, 1 out]
                        n410 = dll-call lib="User32.dll" fn="SetCursorPos"(w1045, w1044) -> ()  [unwired: 6 in, 2 out]
                        n411 = Build Path(base path=w1055, name or relative path="successful_hit.wav") -> (appended path=w1057:path)
                        n412 = call <vilib>:"Play Sound File.vi"("path"=w1057) -> ()  [unwired: 9 in, 2 out]
                        n413 = stacked-sequence {
                          tunnel: w1052 -> [w1064 w1075 w1086 w1096 w1105]
                          tunnel: w1053 -> [_ w1073 _ _ _]
                          tunnel: w1051 -> [_ _ w1084 _ _]
                          tunnel: [_ _ w1082 _ _] -> w1050
                          tunnel: w1049 -> [_ _ w1085 _ _]
                          tunnel: w1048 -> [_ w1068 _ _ _]
                          tunnel: w1041 -> [w1065 _ _ _ _]
                          tunnel: [dbl[][] [] _ _ _ _] -> w1040
                          frame #0 {
                            n414 = call-poly <vilib>:"Write To Spreadsheet File.vi"("append to file? (new file:F)"=TRUE, "2D data"=w1065, "file path (dialog if empty)"=w1064) -> ()  [unwired: 5 in, 1 out]
                          }
                          frame #1 {
                            n415 = Greater?(x=w1068, y=u32 10000 ("element")) -> (0:w1071:bool)
                            n416 = Select(t=1, s=w1071, f=w1068) -> (s? t:f=w1067:i32)
                            n417 = Build Array(w1073, w1067, u32 0 ("element")) -> (w1074:u32[])
                            n418 = call-poly <vilib>:"Write To Spreadsheet File.vi"("append to file? (new file:F)"=TRUE, "1D data"=w1074, "file path (dialog if empty)"=w1075) -> ()  [unwired: 5 in, 1 out]
                          }
                          frame #2 {
                            w1082 = u32 0 ("element")
                            n419 = call "3D_to_Pixels.vi"("Distance_3D"=w1084) -> ("Distance_pixels"=w1083:dbl)  [unwired: 11 in, 3 out]
                            n420 = Decrement(x=w1085) -> (x-1=w1078:u32)
                            n421 = Greater?(x=w1078, y=u32 10000 ("element")) -> (0:w1081:bool)
                            n422 = Select(t=1, s=w1081, f=w1078) -> (s? t:f=w1077:u32)
                            n423 = Build Array(w1083, w1077, w1082) -> (w1088:dbl[])
                            n424 = call-poly <vilib>:"Write To Spreadsheet File.vi"("append to file? (new file:F)"=TRUE, "1D data"=w1088, "file path (dialog if empty)"=w1086) -> ()  [unwired: 5 in, 1 out]
                          }
                          frame #3 {
                            n425 = call "3D_to_Pixels.vi"("X_3D"=-0.8 ("element"), "Y_3D"=-0.8 ("element"), "Z_3D"=-0.8 ("element")) -> ("X_pixels"=w1095:dbl, "Y_pixels"=w1094:dbl, "Z_pixels"=w1093:dbl)  [unwired: 9 in, 1 out]
                            n426 = Build Array(w1095, w1094, w1093) -> (w1089:dbl[])
                            n427 = call-poly <vilib>:"Write To Spreadsheet File.vi"("append to file? (new file:F)"=TRUE, "1D data"=w1089, "file path (dialog if empty)"=w1096) -> ()  [unwired: 5 in, 1 out]
                          }
                          frame #4 {
                            n428 = call "3D_to_Pixels.vi"("X_3D"=0.8 ("element"), "Y_3D"=0.8 ("element"), "Z_3D"=0.8 ("element")) -> ("X_pixels"=w1104:dbl, "Y_pixels"=w1103:dbl, "Z_pixels"=w1102:dbl)  [unwired: 9 in, 1 out]
                            n429 = Build Array(w1104, w1103, w1102) -> (w1098:dbl[])
                            n430 = call-poly <vilib>:"Write To Spreadsheet File.vi"("append to file? (new file:F)"=TRUE, "1D data"=w1098, "file path (dialog if empty)"=w1105) -> ()  [unwired: 5 in, 1 out]
                          }
                        }
                      }
                    }
                  }
                }
              }
              frame 5 {
                n431 = Unbundle(w1115) -> ("X_3D"=w1130:dbl, "Y_3D"=w1129:dbl, "Z"=w1128:dbl)
                n432 = call "3D_Session_Data.vi"("Session"=w1114) -> ("Radius"=w1113:sgl, "min"=w1120:dbl, "max"=w1119:dbl)  [unwired: 8 in]
                n433 = Less Or Equal?(x=w1130, y=w1119) -> (x <= y?=w1126:bool)
                n434 = Greater Or Equal?(x=w1130, y=w1120) -> (x >= y?=w1127:bool)
                n435 = Negate(x=w1119) -> (-x=w1118:dbl)
                n436 = Negate(x=w1120) -> (-x=w1117:dbl)
                n437 = Greater Or Equal?(x=w1129, y=w1118) -> (x >= y?=w1125:bool)
                n438 = Less Or Equal?(x=w1129, y=w1117) -> (x <= y?=w1124:bool)
                n439 = Greater Or Equal?(x=w1128, y=w1118) -> (x >= y?=w1123:bool)
                n440 = Less Or Equal?(x=w1128, y=w1117) -> (x <= y?=w1122:bool)
                n441 = Build Array(w1127, w1126, w1125, w1124, w1123, w1122) -> (w1121:bool[])
                n442 = And Array Elements(Boolean array=w1121) -> (logical AND=w1116:bool)
                n443 = case shown="True" w1116 {
                  tunnel: [T12[] [{"Red"=0.0, "Green"=0.0, "Blue"=0.545, "Alpha"=0.8}, {"Red"=0.0, "Green"=0.0, "Blue"=0.545, "Alpha"=0.8}, {"Red"=0.0, "Green"=0.0, "Blue"=0.545, "Alpha"=0.8}, {"Red"=0.0, "Green"=0.0, "Blue"=0.545, "Alpha"=0.8}, {"Red"=0.0, "Green"=0.0, "Blue"=0.545, "Alpha"=0.8}, {"Red"=0.0, "Green"=1.0, "Blue"=1.0, "Alpha"=0.8}, {"Red"=0.0, "Green"=0.0, "Blue"=0.545, "Alpha"=0.8}, {"Red"=0.0, "Green"=0.0, "Blue"=0.545, "Alpha"=0.8}] ("Array") w1192] -> w1147
                  tunnel: [T11 {"Red"=1.0, "Green"=0.0, "Blue"=0.0, "Alpha"=1.0} ("Color") w1191] -> w1146
                  tunnel: w1145 -> [w1151 w1190]
                  tunnel: w1144 -> [w1160 w1189]
                  tunnel: [w1160 w1188] -> w1143
                  tunnel: w1142 -> [w1159 w1187]
                  tunnel: [w1159 w1186] -> w1141
                  tunnel: w1140 -> [_ w1185]
                  tunnel: w1113 -> [_ w1184]
                  tunnel: [w1158 w1183] -> w1139
                  tunnel: w1138 -> [w1158 w1182]
                  tunnel: w1137 -> [w1155 w1181]
                  tunnel: w1136 -> [w1154 w1180]
                  tunnel: [w1153 w1181] -> w1135
                  tunnel: [w1152 w1179] -> w1134
                  tunnel: w1115 -> [w1150 w1178]
                  tunnel: [w1150 w1177] -> w1133
                  tunnel: w1132 -> [w1149 w1176]
                  tunnel: [w1149 w1175] -> w1131
                  frame False {
                    n444 = case shown="True" w1151 {
                      tunnel: w1155 -> [w1163 w1174]
                      tunnel: [w1162 w1173] -> w1153
                      tunnel: w1154 -> [w1165 w1172]
                      tunnel: [w1164 w1172] -> w1152
                      frame False {
                        n445 = Greater Than 0?(x=w1163) -> (x > 0?=w1166:bool)
                        n446 = case shown="False" w1166 {
                          tunnel: w1165 -> [w1168 w1171]
                          tunnel: [w1168 w1170] -> w1164
                          tunnel: w1163 -> [w1167 _]
                          tunnel: [w1167 0 ("y")] -> w1162
                          frame False {
                          }
                          frame True {
                            n447 = Increment(x=w1171) -> (x+1=w1170:i32)
                          }
                        }
                      }
                      frame True {
                        n448 = Increment(x=w1174) -> (x+1=w1173:i32)
                      }
                    }
                    n449 = Number To Decimal String(number=0) -> (decimal integer string=w1157:string)  [unwired: 1 in]
                    n450 = property on="initial time 2" class="DigNum (strict)"("NumText.Text"=w1157) -> ()  [unwired: 2 in, 2 out]
                  }
                  frame True {
                    n451 = case shown="True" w1190 {
                      tunnel: [T12[] [{"Red"=0.0, "Green"=0.0, "Blue"=0.545, "Alpha"=0.8}, {"Red"=0.0, "Green"=0.0, "Blue"=0.545, "Alpha"=0.8}, {"Red"=0.0, "Green"=0.0, "Blue"=0.545, "Alpha"=0.8}, {"Red"=0.0, "Green"=0.0, "Blue"=0.545, "Alpha"=0.8}, {"Red"=0.0, "Green"=0.0, "Blue"=0.545, "Alpha"=0.8}, {"Red"=0.0, "Green"=0.8, "Blue"=0.0, "Alpha"=0.8}, {"Red"=0.0, "Green"=0.0, "Blue"=0.545, "Alpha"=0.8}, {"Red"=0.0, "Green"=0.0, "Blue"=0.545, "Alpha"=0.8}] ("Array") T12[] [{"Red"=0.0, "Green"=0.0, "Blue"=0.545, "Alpha"=0.8}, {"Red"=0.0, "Green"=0.0, "Blue"=0.545, "Alpha"=0.8}, {"Red"=0.0, "Green"=0.0, "Blue"=0.545, "Alpha"=0.8}, {"Red"=0.0, "Green"=0.0, "Blue"=0.545, "Alpha"=0.8}, {"Red"=0.0, "Green"=0.0, "Blue"=0.545, "Alpha"=0.8}, {"Red"=1.0, "Green"=1.0, "Blue"=0.0, "Alpha"=0.8}, {"Red"=0.0, "Green"=0.0, "Blue"=0.545, "Alpha"=0.8}, {"Red"=0.0, "Green"=0.0, "Blue"=0.545, "Alpha"=0.8}] ("Array")] -> w1192
                      tunnel: [T11 {"Red"=0.0, "Green"=0.8, "Blue"=0.0, "Alpha"=1.0} ("Color") T11 {"Red"=1.0, "Green"=1.0, "Blue"=0.0, "Alpha"=1.0} ("Color")] -> w1191
                      tunnel: w1189 -> [w1203 w1232]
                      tunnel: [w1203 w1231] -> w1188
                      tunnel: w1187 -> [w1202 w1230]
                      tunnel: [w1202 w1229] -> w1186
                      tunnel: w1185 -> [_ w1223]
                      tunnel: w1184 -> [_ w1222]
                      tunnel: [w1197 w1221] -> w1183
                      tunnel: w1182 -> [w1198 w1220]
                      tunnel: w1180 -> [w1196 w1219]
                      tunnel: [w1196 0 ("y")] -> w1179
                      tunnel: w1178 -> [w1195 _]
                      tunnel: [w1195 w1213] -> w1177
                      tunnel: w1176 -> [w1194 w1212]
                      tunnel: [w1194 w1211] -> w1175
                      frame False {
                        n452 = property on="initial time 2" class="DigNum (strict)"() -> ("NumText.Text"=w1200:string)  [unwired: 2 in, 2 out]
                        n453 = Decimal String To Number(string=w1200) -> (number=w1199:i32)  [unwired: 2 in, 1 out]
                        n454 = Equal To 0?(x=w1199) -> (x = 0?=w1201:bool)
                        n455 = case shown="False" w1201 {
                          tunnel: w1198 -> [w1205 w1209]
                          tunnel: [w1205 w1208] -> w1197
                          frame False {
                          }
                          frame True {
                            n456 = Increment(x=w1209) -> (x+1=w1208:u32)
                            n457 = Number To Decimal String(number=1) -> (decimal integer string=w1207:string)  [unwired: 1 in]
                            n458 = property on="initial time 2" class="DigNum (strict)"("NumText.Text"=w1207) -> ()  [unwired: 2 in, 2 out]
                          }
                        }
                      }
                      frame True {
                        w1213 = cluster{dbl, dbl, "y":dbl} {0.8, -0.8, "y"=0.8}
                        n459 = stacked-sequence {
                          seq-local: [w1279 _] -> [_ w1282]
                          tunnel: [w1278 _] -> w1224
                          frame #0 {
                            n460 = property on="initial time" class="DigNum (strict)"() -> ("NumText.Text"=w1281:string)  [unwired: 2 in, 2 out]
                            n461 = Decimal String To Number(string=w1281) -> (number=w1280:i32)  [unwired: 2 in, 1 out]
                            n462 = Tick Count (ms)() -> (millisecond timer value=w1279:u32)
                            n463 = Subtract(x=w1279, y=w1280) -> (x-y=w1278:u32)
                          }
                          frame #1 {
                            n464 = Number To Decimal String(number=w1282) -> (decimal integer string=w1283:string)  [unwired: 1 in]
                            n465 = property on="initial time" class="DigNum (strict)"("NumText.Text"=w1283) -> ()  [unwired: 2 in, 2 out]
                          }
                        }
                        n466 = Increment(x=w1230) -> (x+1=w1229:i32)
                        n467 = Increment(x=w1232) -> (x+1=w1231:i32)
                        n468 = Current VI's Path() -> (path=w1227:path)
                        n469 = Unbundle(w1213) -> (w1217:dbl, w1218:dbl)  [unwired: 1 out]
                        n470 = Strip Path(path=w1227) -> (stripped path=w1226:path)  [unwired: 1 out]
                        n471 = call "3D_to_Screen.vi"("X_3D"=w1217, "Y_3D"=w1218) -> ("X"=w1216:dbl, "Y"=w1215:dbl)  [unwired: 11 in, 1 out]
                        n472 = dll-call lib="User32.dll" fn="SetCursorPos"(w1216, w1215) -> ()  [unwired: 6 in, 2 out]
                        n473 = Build Path(base path=w1226, name or relative path="successful_hit.wav") -> (appended path=w1228:path)
                        n474 = call <vilib>:"Play Sound File.vi"("path"=w1228) -> ()  [unwired: 9 in, 2 out]
                        n475 = stacked-sequence {
                          tunnel: w1223 -> [w1235 w1246 w1257 w1267 w1276]
                          tunnel: w1224 -> [_ w1244 _ _ _]
                          tunnel: w1222 -> [_ _ w1254 _ _]
                          tunnel: [_ _ w1255 _ _] -> w1221
                          tunnel: w1220 -> [_ _ w1256 _ _]
                          tunnel: w1219 -> [_ w1239 _ _ _]
                          tunnel: w1212 -> [w1236 _ _ _ _]
                          tunnel: [dbl[][] [] _ _ _ _] -> w1211
                          frame #0 {
                            n476 = call-poly <vilib>:"Write To Spreadsheet File.vi"("append to file? (new file:F)"=TRUE, "2D data"=w1236, "file path (dialog if empty)"=w1235) -> ()  [unwired: 5 in, 1 out]
                          }
                          frame #1 {
                            n477 = Greater?(x=w1239, y=u32 10000 ("element")) -> (0:w1242:bool)
                            n478 = Select(t=1, s=w1242, f=w1239) -> (s? t:f=w1238:i32)
                            n479 = Build Array(w1244, w1238, u32 0 ("element")) -> (w1245:u32[])
                            n480 = call-poly <vilib>:"Write To Spreadsheet File.vi"("append to file? (new file:F)"=TRUE, "1D data"=w1245, "file path (dialog if empty)"=w1246) -> ()  [unwired: 5 in, 1 out]
                          }
                          frame #2 {
                            w1255 = u32 0 ("element")
                            n481 = call "3D_to_Pixels.vi"("Distance_3D"=w1254) -> ("Distance_pixels"=w1253:dbl)  [unwired: 11 in, 3 out]
                            n482 = Decrement(x=w1256) -> (x-1=w1249:u32)
                            n483 = Greater?(x=w1249, y=u32 10000 ("element")) -> (0:w1252:bool)
                            n484 = Select(t=1, s=w1252, f=w1249) -> (s? t:f=w1248:u32)
                            n485 = Build Array(w1253, w1248, w1255) -> (w1258:dbl[])
                            n486 = call-poly <vilib>:"Write To Spreadsheet File.vi"("append to file? (new file:F)"=TRUE, "1D data"=w1258, "file path (dialog if empty)"=w1257) -> ()  [unwired: 5 in, 1 out]
                          }
                          frame #3 {
                            n487 = call "3D_to_Pixels.vi"("X_3D"=-0.8 ("element"), "Y_3D"=0.8 ("element"), "Z_3D"=0.8 ("element")) -> ("X_pixels"=w1266:dbl, "Y_pixels"=w1265:dbl, "Z_pixels"=w1264:dbl)  [unwired: 9 in, 1 out]
                            n488 = Build Array(w1266, w1265, w1264) -> (w1260:dbl[])
                            n489 = call-poly <vilib>:"Write To Spreadsheet File.vi"("append to file? (new file:F)"=TRUE, "1D data"=w1260, "file path (dialog if empty)"=w1267) -> ()  [unwired: 5 in, 1 out]
                          }
                          frame #4 {
                            n490 = call "3D_to_Pixels.vi"("X_3D"=0.8 ("element"), "Y_3D"=-0.8 ("element"), "Z_3D"=-0.8 ("element")) -> ("X_pixels"=w1275:dbl, "Y_pixels"=w1274:dbl, "Z_pixels"=w1273:dbl)  [unwired: 9 in, 1 out]
                            n491 = Build Array(w1275, w1274, w1273) -> (w1269:dbl[])
                            n492 = call-poly <vilib>:"Write To Spreadsheet File.vi"("append to file? (new file:F)"=TRUE, "1D data"=w1269, "file path (dialog if empty)"=w1276) -> ()  [unwired: 5 in, 1 out]
                          }
                        }
                      }
                    }
                  }
                }
              }
              frame 6 {
                n493 = Unbundle(w1285) -> ("X_3D"=w1301:dbl, "Y_3D"=w1300:dbl, "Z"=w1299:dbl)
                n494 = call "3D_Session_Data.vi"("Session"=w1286) -> ("Radius"=w1284:sgl, "min"=w1291:dbl, "max"=w1290:dbl)  [unwired: 8 in]
                n495 = Less Or Equal?(x=w1300, y=w1290) -> (x <= y?=w1295:bool)
                n496 = Greater Or Equal?(x=w1300, y=w1291) -> (x >= y?=w1296:bool)
                n497 = Negate(x=w1290) -> (-x=w1289:dbl)
                n498 = Negate(x=w1291) -> (-x=w1288:dbl)
                n499 = Greater Or Equal?(x=w1301, y=w1289) -> (x >= y?=w1298:bool)
                n500 = Less Or Equal?(x=w1301, y=w1288) -> (x <= y?=w1297:bool)
                n501 = Greater Or Equal?(x=w1299, y=w1289) -> (x >= y?=w1294:bool)
                n502 = Less Or Equal?(x=w1299, y=w1288) -> (x <= y?=w1293:bool)
                n503 = Build Array(w1298, w1297, w1296, w1295, w1294, w1293) -> (w1292:bool[])
                n504 = And Array Elements(Boolean array=w1292) -> (logical AND=w1287:bool)
                n505 = case shown="True" w1287 {
                  tunnel: [T12[] [{"Red"=0.0, "Green"=0.0, "Blue"=0.545, "Alpha"=0.8}, {"Red"=0.0, "Green"=0.0, "Blue"=0.545, "Alpha"=0.8}, {"Red"=0.0, "Green"=0.0, "Blue"=0.545, "Alpha"=0.8}, {"Red"=0.0, "Green"=0.0, "Blue"=0.545, "Alpha"=0.8}, {"Red"=0.0, "Green"=0.0, "Blue"=0.545, "Alpha"=0.8}, {"Red"=0.0, "Green"=0.0, "Blue"=0.545, "Alpha"=0.8}, {"Red"=0.0, "Green"=1.0, "Blue"=1.0, "Alpha"=0.8}, {"Red"=0.0, "Green"=0.0, "Blue"=0.545, "Alpha"=0.8}] ("Array") w1363] -> w1318
                  tunnel: [T11 {"Red"=1.0, "Green"=0.0, "Blue"=0.0, "Alpha"=1.0} ("Color") w1362] -> w1317
                  tunnel: w1316 -> [w1326 w1361]
                  tunnel: w1315 -> [w1331 w1360]
                  tunnel: [w1331 w1359] -> w1314
                  tunnel: w1313 -> [w1330 w1358]
                  tunnel: [w1330 w1357] -> w1312
                  tunnel: w1311 -> [_ w1356]
                  tunnel: w1284 -> [_ w1355]
                  tunnel: [w1329 w1354] -> w1310
                  tunnel: w1309 -> [w1329 w1353]
                  tunnel: w1308 -> [w1325 w1352]
                  tunnel: w1307 -> [w1324 w1351]
                  tunnel: [w1323 w1352] -> w1306
                  tunnel: [w1322 w1350] -> w1305
                  tunnel: w1285 -> [w1321 w1349]
                  tunnel: [w1321 w1348] -> w1304
                  tunnel: w1303 -> [w1320 w1347]
                  tunnel: [w1320 w1346] -> w1302
                  frame False {
                    n506 = case shown="False" w1326 {
                      tunnel: w1325 -> [w1334 w1345]
                      tunnel: [w1333 w1344] -> w1323
                      tunnel: w1324 -> [w1336 w1343]
                      tunnel: [w1335 w1343] -> w1322
                      frame False {
                        n507 = Greater Than 0?(x=w1334) -> (x > 0?=w1337:bool)
                        n508 = case shown="True" w1337 {
                          tunnel: w1336 -> [w1339 w1342]
                          tunnel: [w1339 w1341] -> w1335
                          tunnel: w1334 -> [w1338 _]
                          tunnel: [w1338 0 ("y")] -> w1333
                          frame False {
                          }
                          frame True {
                            n509 = Increment(x=w1342) -> (x+1=w1341:i32)
                          }
                        }
                      }
                      frame True {
                        n510 = Increment(x=w1345) -> (x+1=w1344:i32)
                      }
                    }
                    n511 = Number To Decimal String(number=0) -> (decimal integer string=w1328:string)  [unwired: 1 in]
                    n512 = property on="initial time 2" class="DigNum (strict)"("NumText.Text"=w1328) -> ()  [unwired: 2 in, 2 out]
                  }
                  frame True {
                    n513 = case shown="True" w1361 {
                      tunnel: [T12[] [{"Red"=0.0, "Green"=0.0, "Blue"=0.545, "Alpha"=0.8}, {"Red"=0.0, "Green"=0.0, "Blue"=0.545, "Alpha"=0.8}, {"Red"=0.0, "Green"=0.0, "Blue"=0.545, "Alpha"=0.8}, {"Red"=0.0, "Green"=0.0, "Blue"=0.545, "Alpha"=0.8}, {"Red"=0.0, "Green"=0.0, "Blue"=0.545, "Alpha"=0.8}, {"Red"=0.0, "Green"=0.0, "Blue"=0.545, "Alpha"=0.8}, {"Red"=0.0, "Green"=0.8, "Blue"=0.0, "Alpha"=0.8}, {"Red"=0.0, "Green"=0.0, "Blue"=0.545, "Alpha"=0.8}] ("Array") T12[] [{"Red"=0.0, "Green"=0.0, "Blue"=0.545, "Alpha"=0.8}, {"Red"=0.0, "Green"=0.0, "Blue"=0.545, "Alpha"=0.8}, {"Red"=0.0, "Green"=0.0, "Blue"=0.545, "Alpha"=0.8}, {"Red"=0.0, "Green"=0.0, "Blue"=0.545, "Alpha"=0.8}, {"Red"=0.0, "Green"=0.0, "Blue"=0.545, "Alpha"=0.8}, {"Red"=0.0, "Green"=0.0, "Blue"=0.545, "Alpha"=0.8}, {"Red"=1.0, "Green"=1.0, "Blue"=0.0, "Alpha"=0.8}, {"Red"=0.0, "Green"=0.0, "Blue"=0.545, "Alpha"=0.8}] ("Array")] -> w1363
                      tunnel: [T11 {"Red"=0.0, "Green"=0.8, "Blue"=0.0, "Alpha"=1.0} ("Color") T11 {"Red"=1.0, "Green"=1.0, "Blue"=0.0, "Alpha"=1.0} ("Color")] -> w1362
                      tunnel: w1360 -> [w1374 w1403]
                      tunnel: [w1374 w1402] -> w1359
                      tunnel: w1358 -> [w1373 w1401]
                      tunnel: [w1373 w1400] -> w1357
                      tunnel: w1356 -> [_ w1394]
                      tunnel: w1355 -> [_ w1393]
                      tunnel: [w1369 w1392] -> w1354
                      tunnel: w1353 -> [w1368 w1391]
                      tunnel: w1351 -> [w1367 w1390]
                      tunnel: [w1367 0 ("y")] -> w1350
                      tunnel: w1349 -> [w1366 _]
                      tunnel: [w1366 w1384] -> w1348
                      tunnel: w1347 -> [w1365 w1383]
                      tunnel: [w1365 w1382] -> w1346
                      frame False {
                        n514 = property on="initial time 2" class="DigNum (strict)"() -> ("NumText.Text"=w1371:string)  [unwired: 2 in, 2 out]
                        n515 = Decimal String To Number(string=w1371) -> (number=w1370:i32)  [unwired: 2 in, 1 out]
                        n516 = Equal To 0?(x=w1370) -> (x = 0?=w1372:bool)
                        n517 = case shown="False" w1372 {
                          tunnel: w1368 -> [w1376 w1380]
                          tunnel: [w1376 w1379] -> w1369
                          frame False {
                          }
                          frame True {
                            n518 = Increment(x=w1380) -> (x+1=w1379:u32)
                            n519 = Number To Decimal String(number=1) -> (decimal integer string=w1378:string)  [unwired: 1 in]
                            n520 = property on="initial time 2" class="DigNum (strict)"("NumText.Text"=w1378) -> ()  [unwired: 2 in, 2 out]
                          }
                        }
                      }
                      frame True {
                        w1384 = cluster{dbl, dbl, "y":dbl} {0.8, 0.8, "y"=-0.8}
                        n521 = stacked-sequence {
                          seq-local: [w1450 _] -> [_ w1453]
                          tunnel: [w1449 _] -> w1395
                          frame #0 {
                            n522 = property on="initial time" class="DigNum (strict)"() -> ("NumText.Text"=w1452:string)  [unwired: 2 in, 2 out]
                            n523 = Decimal String To Number(string=w1452) -> (number=w1451:i32)  [unwired: 2 in, 1 out]
                            n524 = Tick Count (ms)() -> (millisecond timer value=w1450:u32)
                            n525 = Subtract(x=w1450, y=w1451) -> (x-y=w1449:u32)
                          }
                          frame #1 {
                            n526 = Number To Decimal String(number=w1453) -> (decimal integer string=w1454:string)  [unwired: 1 in]
                            n527 = property on="initial time" class="DigNum (strict)"("NumText.Text"=w1454) -> ()  [unwired: 2 in, 2 out]
                          }
                        }
                        n528 = Increment(x=w1401) -> (x+1=w1400:i32)
                        n529 = Increment(x=w1403) -> (x+1=w1402:i32)
                        n530 = Current VI's Path() -> (path=w1398:path)
                        n531 = Unbundle(w1384) -> (w1388:dbl, w1389:dbl)  [unwired: 1 out]
                        n532 = Strip Path(path=w1398) -> (stripped path=w1397:path)  [unwired: 1 out]
                        n533 = call "3D_to_Screen.vi"("X_3D"=w1388, "Y_3D"=w1389) -> ("X"=w1387:dbl, "Y"=w1386:dbl)  [unwired: 11 in, 1 out]
                        n534 = dll-call lib="User32.dll" fn="SetCursorPos"(w1387, w1386) -> ()  [unwired: 6 in, 2 out]
                        n535 = Build Path(base path=w1397, name or relative path="successful_hit.wav") -> (appended path=w1399:path)
                        n536 = call <vilib>:"Play Sound File.vi"("path"=w1399) -> ()  [unwired: 9 in, 2 out]
                        n537 = stacked-sequence {
                          tunnel: w1394 -> [w1406 w1417 w1428 w1438 w1447]
                          tunnel: w1395 -> [_ w1415 _ _ _]
                          tunnel: w1393 -> [_ _ w1425 _ _]
                          tunnel: [_ _ w1426 _ _] -> w1392
                          tunnel: w1391 -> [_ _ w1427 _ _]
                          tunnel: w1390 -> [_ w1410 _ _ _]
                          tunnel: w1383 -> [w1407 _ _ _ _]
                          tunnel: [dbl[][] [] _ _ _ _] -> w1382
                          frame #0 {
                            n538 = call-poly <vilib>:"Write To Spreadsheet File.vi"("append to file? (new file:F)"=TRUE, "2D data"=w1407, "file path (dialog if empty)"=w1406) -> ()  [unwired: 5 in, 1 out]
                          }
                          frame #1 {
                            n539 = Greater?(x=w1410, y=u32 10000 ("element")) -> (0:w1413:bool)
                            n540 = Select(t=1, s=w1413, f=w1410) -> (s? t:f=w1409:i32)
                            n541 = Build Array(w1415, w1409, u32 0 ("element")) -> (w1416:u32[])
                            n542 = call-poly <vilib>:"Write To Spreadsheet File.vi"("append to file? (new file:F)"=TRUE, "1D data"=w1416, "file path (dialog if empty)"=w1417) -> ()  [unwired: 5 in, 1 out]
                          }
                          frame #2 {
                            w1426 = u32 0 ("element")
                            n543 = call "3D_to_Pixels.vi"("Distance_3D"=w1425) -> ("Distance_pixels"=w1424:dbl)  [unwired: 11 in, 3 out]
                            n544 = Decrement(x=w1427) -> (x-1=w1420:u32)
                            n545 = Greater?(x=w1420, y=u32 10000 ("element")) -> (0:w1423:bool)
                            n546 = Select(t=1, s=w1423, f=w1420) -> (s? t:f=w1419:u32)
                            n547 = Build Array(w1424, w1419, w1426) -> (w1429:dbl[])
                            n548 = call-poly <vilib>:"Write To Spreadsheet File.vi"("append to file? (new file:F)"=TRUE, "1D data"=w1429, "file path (dialog if empty)"=w1428) -> ()  [unwired: 5 in, 1 out]
                          }
                          frame #3 {
                            n549 = call "3D_to_Pixels.vi"("X_3D"=0.8 ("element"), "Y_3D"=-0.8 ("element"), "Z_3D"=0.8 ("element")) -> ("X_pixels"=w1437:dbl, "Y_pixels"=w1436:dbl, "Z_pixels"=w1435:dbl)  [unwired: 9 in, 1 out]
                            n550 = Build Array(w1437, w1436, w1435) -> (w1431:dbl[])
                            n551 = call-poly <vilib>:"Write To Spreadsheet File.vi"("append to file? (new file:F)"=TRUE, "1D data"=w1431, "file path (dialog if empty)"=w1438) -> ()  [unwired: 5 in, 1 out]
                          }
                          frame #4 {
                            n552 = call "3D_to_Pixels.vi"("X_3D"=-0.8 ("element"), "Y_3D"=0.8 ("element"), "Z_3D"=-0.8 ("element")) -> ("X_pixels"=w1446:dbl, "Y_pixels"=w1445:dbl, "Z_pixels"=w1444:dbl)  [unwired: 9 in, 1 out]
                            n553 = Build Array(w1446, w1445, w1444) -> (w1440:dbl[])
                            n554 = call-poly <vilib>:"Write To Spreadsheet File.vi"("append to file? (new file:F)"=TRUE, "1D data"=w1440, "file path (dialog if empty)"=w1447) -> ()  [unwired: 5 in, 1 out]
                          }
                        }
                      }
                    }
                  }
                }
              }
              frame 7, Default {
                n555 = Unbundle(w1457) -> ("X_3D"=w1472:dbl, "Y_3D"=w1471:dbl, "Z"=w1470:dbl)
                n556 = call "3D_Session_Data.vi"("Session"=w1456) -> ("Radius"=w1455:sgl, "min"=w1460:dbl, "max"=w1459:dbl)  [unwired: 8 in]
                n557 = Less Or Equal?(x=w1470, y=w1459) -> (x <= y?=w1464:bool)
                n558 = Greater Or Equal?(x=w1470, y=w1460) -> (x >= y?=w1465:bool)
                n559 = Negate(x=w1459) -> (-x=w1462:dbl)
                n560 = Negate(x=w1460) -> (-x=w1461:dbl)
                n561 = Greater Or Equal?(x=w1472, y=w1462) -> (x >= y?=w1469:bool)
                n562 = Less Or Equal?(x=w1472, y=w1461) -> (x <= y?=w1468:bool)
                n563 = Greater Or Equal?(x=w1471, y=w1462) -> (x >= y?=w1467:bool)
                n564 = Less Or Equal?(x=w1471, y=w1461) -> (x <= y?=w1466:bool)
                n565 = Build Array(w1469, w1468, w1467, w1466, w1465, w1464) -> (w1463:bool[])
                n566 = And Array Elements(Boolean array=w1463) -> (logical AND=w1458:bool)
                n567 = case shown="True" w1458 {
                  tunnel: [T12[] [{"Red"=0.0, "Green"=0.0, "Blue"=0.545, "Alpha"=0.8}, {"Red"=0.0, "Green"=1.0, "Blue"=1.0, "Alpha"=0.8}, {"Red"=0.0, "Green"=0.0, "Blue"=0.545, "Alpha"=0.8}, {"Red"=0.0, "Green"=0.0, "Blue"=0.545, "Alpha"=0.8}, {"Red"=0.0, "Green"=0.0, "Blue"=0.545, "Alpha"=0.8}, {"Red"=0.0, "Green"=0.0, "Blue"=0.545, "Alpha"=0.8}, {"Red"=0.0, "Green"=0.0, "Blue"=0.545, "Alpha"=0.8}, {"Red"=0.0, "Green"=0.0, "Blue"=0.545, "Alpha"=0.8}] ("Array") w1534] -> w1489
                  tunnel: [T11 {"Red"=1.0, "Green"=0.0, "Blue"=0.0, "Alpha"=1.0} ("Color") w1533] -> w1488
                  tunnel: w1487 -> [w1497 w1532]
                  tunnel: w1486 -> [w1502 w1531]
                  tunnel: [w1502 w1530] -> w1485
                  tunnel: w1484 -> [w1501 w1529]
                  tunnel: [w1501 w1528] -> w1483
                  tunnel: w1482 -> [_ w1527]
                  tunnel: w1455 -> [_ w1526]
                  tunnel: w1481 -> [w1500 w1525]
                  tunnel: [w1500 w1524] -> w1480
                  tunnel: w1479 -> [w1496 w1523]
                  tunnel: w1478 -> [w1495 w1522]
                  tunnel: [w1494 w1521] -> w1477
                  tunnel: [w1493 w1523] -> w1476
                  tunnel: w1457 -> [w1492 w1520]
                  tunnel: [w1492 w1519] -> w1475
                  tunnel: w1474 -> [w1491 w1518]
                  tunnel: [w1491 w1517] -> w1473
                  frame False {
                    n568 = case shown="False" w1497 {
                      tunnel: w1496 -> [w1505 w1516]
                      tunnel: [w1504 w1515] -> w1493
                      tunnel: w1495 -> [w1507 w1514]
                      tunnel: [w1506 w1514] -> w1494
                      frame False {
                        n569 = Greater Than 0?(x=w1505) -> (x > 0?=w1508:bool)
                        n570 = case shown="True" w1508 {
                          tunnel: w1507 -> [w1510 w1513]
                          tunnel: [w1510 w1512] -> w1506
                          tunnel: w1505 -> [w1509 _]
                          tunnel: [w1509 0 ("y")] -> w1504
                          frame False {
                          }
                          frame True {
                            n571 = Increment(x=w1513) -> (x+1=w1512:i32)
                          }
                        }
                      }
                      frame True {
                        n572 = Increment(x=w1516) -> (x+1=w1515:i32)
                      }
                    }
                    n573 = Number To Decimal String(number=0) -> (decimal integer string=w1499:string)  [unwired: 1 in]
                    n574 = property on="initial time 2" class="DigNum (strict)"("NumText.Text"=w1499) -> ()  [unwired: 2 in, 2 out]
                  }
                  frame True {
                    n575 = case shown="True" w1532 {
                      tunnel: [T12[] [{"Red"=0.0, "Green"=0.0, "Blue"=0.545, "Alpha"=0.8}, {"Red"=0.0, "Green"=0.8, "Blue"=0.0, "Alpha"=0.8}, {"Red"=0.0, "Green"=0.0, "Blue"=0.545, "Alpha"=0.8}, {"Red"=0.0, "Green"=0.0, "Blue"=0.545, "Alpha"=0.8}, {"Red"=0.0, "Green"=0.0, "Blue"=0.545, "Alpha"=0.8}, {"Red"=0.0, "Green"=0.0, "Blue"=0.545, "Alpha"=0.8}, {"Red"=0.0, "Green"=0.0, "Blue"=0.545, "Alpha"=0.8}, {"Red"=0.0, "Green"=0.0, "Blue"=0.545, "Alpha"=0.8}] ("Array") T12[] [{"Red"=0.0, "Green"=0.0, "Blue"=0.545, "Alpha"=0.8}, {"Red"=1.0, "Green"=1.0, "Blue"=0.0, "Alpha"=0.8}, {"Red"=0.0, "Green"=0.0, "Blue"=0.545, "Alpha"=0.8}, {"Red"=0.0, "Green"=0.0, "Blue"=0.545, "Alpha"=0.8}, {"Red"=0.0, "Green"=0.0, "Blue"=0.545, "Alpha"=0.8}, {"Red"=0.0, "Green"=0.0, "Blue"=0.545, "Alpha"=0.8}, {"Red"=0.0, "Green"=0.0, "Blue"=0.545, "Alpha"=0.8}, {"Red"=0.0, "Green"=0.0, "Blue"=0.545, "Alpha"=0.8}] ("Array")] -> w1534
                      tunnel: [T11 {"Red"=0.0, "Green"=0.8, "Blue"=0.0, "Alpha"=1.0} ("Color") T11 {"Red"=1.0, "Green"=1.0, "Blue"=0.0, "Alpha"=1.0} ("Color")] -> w1533
                      tunnel: w1531 -> [w1545 w1574]
                      tunnel: [w1545 w1573] -> w1530
                      tunnel: w1529 -> [w1544 w1572]
                      tunnel: [w1544 w1571] -> w1528
                      tunnel: w1527 -> [_ w1565]
                      tunnel: w1526 -> [_ w1564]
                      tunnel: w1525 -> [w1539 w1563]
                      tunnel: [w1540 w1562] -> w1524
                      tunnel: w1522 -> [w1538 w1561]
                      tunnel: [w1538 0 ("x")] -> w1521
                      tunnel: w1520 -> [w1537 _]
                      tunnel: [w1537 w1555] -> w1519
                      tunnel: w1518 -> [w1536 w1554]
                      tunnel: [w1536 w1553] -> w1517
                      frame False {
                        n576 = property on="initial time 2" class="DigNum (strict)"() -> ("NumText.Text"=w1542:string)  [unwired: 2 in, 2 out]
                        n577 = Decimal String To Number(string=w1542) -> (number=w1541:i32)  [unwired: 2 in, 1 out]
                        n578 = Equal To 0?(x=w1541) -> (x = 0?=w1543:bool)
                        n579 = case shown="False" w1543 {
                          tunnel: w1539 -> [w1547 w1551]
                          tunnel: [w1547 w1550] -> w1540
                          frame False {
                          }
                          frame True {
                            n580 = Increment(x=w1551) -> (x+1=w1550:u32)
                            n581 = Number To Decimal String(number=1) -> (decimal integer string=w1549:string)  [unwired: 1 in]
                            n582 = property on="initial time 2" class="DigNum (strict)"("NumText.Text"=w1549) -> ()  [unwired: 2 in, 2 out]
                          }
                        }
                      }
                      frame True {
                        w1555 = cluster{dbl, dbl, "y":dbl} {-0.8, -0.8, "y"=0.8}
                        n583 = stacked-sequence {
                          seq-local: [w1621 _] -> [_ w1624]
                          tunnel: [w1620 _] -> w1566
                          frame #0 {
                            n584 = property on="initial time" class="DigNum (strict)"() -> ("NumText.Text"=w1623:string)  [unwired: 2 in, 2 out]
                            n585 = Decimal String To Number(string=w1623) -> (number=w1622:i32)  [unwired: 2 in, 1 out]
                            n586 = Tick Count (ms)() -> (millisecond timer value=w1621:u32)
                            n587 = Subtract(x=w1621, y=w1622) -> (x-y=w1620:u32)
                          }
                          frame #1 {
                            n588 = Number To Decimal String(number=w1624) -> (decimal integer string=w1625:string)  [unwired: 1 in]
                            n589 = property on="initial time" class="DigNum (strict)"("NumText.Text"=w1625) -> ()  [unwired: 2 in, 2 out]
                          }
                        }
                        n590 = Increment(x=w1572) -> (x+1=w1571:i32)
                        n591 = Increment(x=w1574) -> (x+1=w1573:i32)
                        n592 = Current VI's Path() -> (path=w1569:path)
                        n593 = Unbundle(w1555) -> (w1559:dbl, w1560:dbl)  [unwired: 1 out]
                        n594 = Strip Path(path=w1569) -> (stripped path=w1568:path)  [unwired: 1 out]
                        n595 = call "3D_to_Screen.vi"("X_3D"=w1559, "Y_3D"=w1560) -> ("X"=w1558:dbl, "Y"=w1557:dbl)  [unwired: 11 in, 1 out]
                        n596 = dll-call lib="User32.dll" fn="SetCursorPos"(w1558, w1557) -> ()  [unwired: 6 in, 2 out]
                        n597 = Build Path(base path=w1568, name or relative path="successful_hit.wav") -> (appended path=w1570:path)
                        n598 = call <vilib>:"Play Sound File.vi"("path"=w1570) -> ()  [unwired: 9 in, 2 out]
                        n599 = stacked-sequence {
                          tunnel: w1565 -> [w1578 w1588 w1599 w1609 w1618]
                          tunnel: w1566 -> [_ w1586 _ _ _]
                          tunnel: w1564 -> [_ _ w1596 _ _]
                          tunnel: w1563 -> [_ _ w1598 _ _]
                          tunnel: [_ _ w1597 _ _] -> w1562
                          tunnel: w1561 -> [_ w1581 _ _ _]
                          tunnel: w1554 -> [w1577 _ _ _ _]
                          tunnel: [dbl[][] [] _ _ _ _] -> w1553
                          frame #0 {
                            n600 = call-poly <vilib>:"Write To Spreadsheet File.vi"("append to file? (new file:F)"=TRUE, "2D data"=w1577, "file path (dialog if empty)"=w1578) -> ()  [unwired: 5 in, 1 out]
                          }
                          frame #1 {
                            n601 = Greater?(x=w1581, y=u32 10000 ("element")) -> (0:w1584:bool)
                            n602 = Select(t=1, s=w1584, f=w1581) -> (s? t:f=w1580:i32)
                            n603 = Build Array(w1586, w1580, u32 0 ("element")) -> (w1587:u32[])
                            n604 = call-poly <vilib>:"Write To Spreadsheet File.vi"("append to file? (new file:F)"=TRUE, "1D data"=w1587, "file path (dialog if empty)"=w1588) -> ()  [unwired: 5 in, 1 out]
                          }
                          frame #2 {
                            w1597 = u32 0 ("element")
                            n605 = call "3D_to_Pixels.vi"("Distance_3D"=w1596) -> ("Distance_pixels"=w1595:dbl)  [unwired: 11 in, 3 out]
                            n606 = Decrement(x=w1598) -> (x-1=w1591:u32)
                            n607 = Greater?(x=w1591, y=u32 10000 ("element")) -> (0:w1594:bool)
                            n608 = Select(t=1, s=w1594, f=w1591) -> (s? t:f=w1590:u32)
                            n609 = Build Array(w1595, w1590, w1597) -> (w1600:dbl[])
                            n610 = call-poly <vilib>:"Write To Spreadsheet File.vi"("append to file? (new file:F)"=TRUE, "1D data"=w1600, "file path (dialog if empty)"=w1599) -> ()  [unwired: 5 in, 1 out]
                          }
                          frame #3 {
                            n611 = call "3D_to_Pixels.vi"("X_3D"=0.8 ("element"), "Y_3D"=0.8 ("element"), "Z_3D"=-0.8 ("element")) -> ("X_pixels"=w1608:dbl, "Y_pixels"=w1607:dbl, "Z_pixels"=w1606:dbl)  [unwired: 9 in, 1 out]
                            n612 = Build Array(w1608, w1607, w1606) -> (w1605:dbl[])
                            n613 = call-poly <vilib>:"Write To Spreadsheet File.vi"("append to file? (new file:F)"=TRUE, "1D data"=w1605, "file path (dialog if empty)"=w1609) -> ()  [unwired: 5 in, 1 out]
                          }
                          frame #4 {
                            n614 = call "3D_to_Pixels.vi"("X_3D"=-0.8 ("element"), "Y_3D"=-0.8 ("element"), "Z_3D"=0.8 ("element")) -> ("X_pixels"=w1617:dbl, "Y_pixels"=w1616:dbl, "Z_pixels"=w1615:dbl)  [unwired: 9 in, 1 out]
                            n615 = Build Array(w1617, w1616, w1615) -> (w1614:dbl[])
                            n616 = call-poly <vilib>:"Write To Spreadsheet File.vi"("append to file? (new file:F)"=TRUE, "1D data"=w1614, "file path (dialog if empty)"=w1618) -> ()  [unwired: 5 in, 1 out]
                          }
                        }
                      }
                    }
                  }
                }
              }
            }
          }
        }
        n617 = call <vilib>:"Set Translation.vi"("Translation"=w119, "Scene Object"=w180) -> ("Translated Object"=w178:refnum<vi>)  [unwired: 8 in, 1 out]
        n618 = Unbundle(w119) -> ("y"=w118:dbl)  [unwired: 2 out]
        n619 = for {
          tunnel: w177 -> [w199] mode=indexing
          tunnel: w176 -> [w202] mode=indexing
          tunnel: w174 -> [w201]
          tunnel: w173 -> [w200] mode=indexing
          n620 = property class="SceneObject"(reference=w199, "Material.Diffuse"=w202) -> ()  [unwired: 1 in, 2 out]
          n621 = property class="SceneSphere"(reference=w200, "Radius"=w201) -> ()  [unwired: 1 in, 2 out]
        }
        n622 = property class="SceneSphere"(reference=w175, "Radius"=w174) -> ()  [unwired: 1 in, 2 out]
        n623 = property class="SceneObject"(reference=w178, "Material.Diffuse"=w179) -> ()  [unwired: 1 in, 2 out]
        n624 = node-c288() -> ()  [unwired: 1 in, 1 out]
        "3D Picture" <- w181
      }
      n625 = node-c288(w107) -> ()  [unwired: 1 out]
    }
    frame #2 {
      n626 = call "Time Delay2"() -> ()  [unwired: 11 in, 1 out]
    }
  }
  n627 = call-poly <vilib>:"Close Input Device.vi"("device ID"=w26) -> ()  [unwired: 1 in, 9 out]
  n628 = property class="VI"(reference=w4, error in=w3, "Front Panel Window:Open"=TRUE) -> (reference out=w7:refnum<vi>, error out=w6:errorcluster)
  n629 = Close Reference(reference=w7, error in (no error)=w6) -> ()  [unwired: 1 out]
